vi "Visualize_R&V_Refactored.vi"() -> ()   [LabVIEW 2016]
uses:
  <vilib>/Utility/miscctls.llb/LVPointDoubleTypeDef.ctl
  subVI/DataVIS_StateWire.ctl
panel:
  in  "Decimate Controls 2":T1={"X Low"=-0.1, "X High"=0.1, "X Step"=4e-05, "Voffset -2T"=0.0} {"X Step" format="%#_6p"; "X High" format="%#_6p"; "X Low" format="%#_6p"}
  in  "Decimate Controls":T1={"X Low"=-0.1, "X High"=0.1, "X Step"=4e-05, "Voffset -2T"=0.0} {"X Step" format="%#_6p"; "X High" format="%#_6p"; "X Low" format="%#_6p"}
  in  "Voffset - 2T":dbl format="%#_13g"
  out "Vsd vs Vsg":cluster{dbl[], dbl[]}(graph)
  out "Intensity Graph 12":dbl[][](graph)
  in  "file path (use dialog) 2":path=path "B:/SketchSET/SA03008H.20180718/processed/decimated_21-BG+SG_Sweep+OVERNIGHT"
  out "slowest 2":dbl=4.2894631624221803e-07
  out "Scan names 3":string[](array[string])=["DSA_Vsg1", "B", "B"]
  in  "stop 2":bool
  out "Vfast index":dbl=3.0
  out "Vslow index":i32
  out "side points 4Ttemp 2":i32=8
  out "side points 2Ttemp 2":i32=12
  in  "side points 4T 3":i32=8
  in  "side points 2T 3":i32=12
  in  "Fit Points 3":dbl=10.0
  in  "T/B     third axis 2":bool
  in  "color scale 2":u32[](array[colorbox])=[16711680, 16772608, 6618880, 3381759, 16860, 10420479]
  in  "Voffset -2T 2":dbl=2e-05 format="%#_6p"
  in  "Voffset-4T 2":dbl=-5e-05 format="%#_4p"
  in  "Filter retrieved data?":bool=TRUE
  in  "Field/Temperature 2":i32(slide) min=0 max=36 step=1
  in  "Generate (T) or Visualize (F)":bool
  in  "Tab Control":T2(tab)=enum."3D"
  out "Comments":string="      #Vslow/#Vfast/# of IV curves/BT offset/#discarded IV curves/Manual offset:\n /101/41/1/0/0/0    \n#of fields: 1    \nField period 1 \nDecimate point 10.000000 \nScan names \nDSA_Vsg1\nB\nB \n IGOR\nX// Date: 7/19/2018 7:21 AM\nX// SA03008H\nX// \nX// Source 2 Drain 28 (lockin 1 and 7)\nX// Slow sweeping BG -5 to 5 inc. 0.1V \nX// Fast sweep SG -1 to 1 inc. 0.05V\n\nX// DSA_Vsg1=1.000000\n\nX// \nX// B= 0.000000\n\n\n\n\n\n\n\n\n\n\n\n\n\n\n\n\n\n\n\n\n\n\n\n\n\n\n\n\n\n\n\n\n\n\n\n\n\n\n\n\nX \nX Display/R 'time.SA03008H.20180718.004140'\nX AppendToGraph 'temp.SA03008H.20180718.004140'\nX AppendToGraph 'B.SA03008H.20180718.004140'\nX AppendToGraph 'Vsource.SA03008H.20180718.004140'\nX AppendToGraph 'Lockin0.SA03008H.20180718.004140'\nX AppendToGraph 'Lockin1.SA03008H.20180718.004140'\nX AppendToGraph 'Lockin2.SA03008H.20180718.004140'\nX AppendToGraph 'Lockin3.SA03008H.20180718.004140'\nX AppendToGraph 'Lockin4.SA03008H.20180718.004140'\nX AppendToGraph 'Lockin5.SA03008H.20180718.004140'\nX AppendToGraph 'B_rate.SA03008H.20180718.004140'\nX AppendToGraph 'DC0.SA03008H.20180718.004140'\nX AppendToGraph 'DC1.SA03008H.20180718.004140'\nX AppendToGraph 'DC2.SA03008H.20180718.004140'\nX AppendToGraph 'DC3.SA03008H.20180718.004140'\nX AppendToGraph 'DC4.SA03008H.20180718.004140'\nX AppendToGraph 'DC5.SA03008H.20180718.004140'\nX AppendToGraph 'DC6.SA03008H.20180718.004140'\nX AppendToGraph 'DC7.SA03008H.20180718.004140'\nX Label bottom \"x label\"\nX Label left \"y label\"\nX ModifyGraph rgb('time.SA03008H.20180718.004140')=(65280,0,0)\nX ModifyGraph rgb('temp.SA03008H.20180718.004140')=(65280,18432,0)\nX ModifyGraph rgb('B.SA03008H.20180718.004140')=(65280,36864,0)\nX ModifyGraph rgb('Vsource.SA03008H.20180718.004140')=(65280,55296,0)\nX ModifyGraph rgb('Lockin0.SA03008H.20180718.004140')=(57344,65280,0)\nX ModifyGraph rgb('Lockin1.SA03008H.20180718.004140')=(37376,65280,0)\nX ModifyGraph rgb('Lockin2.SA03008H.20180718.004140')=(18944,65280,0)\nX ModifyGraph rgb('Lockin3.SA03008H.20180718.004140')=(512,65280,0)\nX ModifyGraph rgb('Lockin4.SA03008H.20180718.004140')=(0,65280,17920)\nX ModifyGraph rgb('Lockin5.SA03008H.20180718.004140')=(0,65280,36352)\nX ModifyGraph rgb('B_rate.SA03008H.20180718.004140')=(0,65280,54784)\nX ModifyGraph rgb('DC0.SA03008H.20180718.004140')=(0,57856,65280)\nX ModifyGraph rgb('DC1.SA03008H.20180718.004140')=(0,39424,65280)\nX ModifyGraph rgb('DC2.SA03008H.20180718.004140')=(0,20992,65280)\nX ModifyGraph rgb('DC3.SA03008H.20180718.004140')=(0,2560,65280)\nX ModifyGraph rgb('DC4.SA03008H.20180718.004140')=(17408,0,65280)\nX ModifyGraph rgb('DC5.SA03008H.20180718.004140')=(35840,0,65280)\nX ModifyGraph rgb('DC6.SA03008H.20180718.004140')=(54272,0,65280)\nX ModifyGraph rgb('DC7.SA03008H.20180718.004140')=(65280,0,58368)\nX Legend/C/N=text0/J \"\\\\s('time.SA03008H.20180718.004140') time\\r\\\\s('temp.SA03008H.20180718.004140') temp\\r\\\\s('B.SA03008H.20180718.004140') B\\r\\\\s('Vsource.SA03008H.20180718.004140') Vsource\\r\\\\s('Lockin0.SA03008H.20180718.004140') Lockin0\\r\\\\s('Lockin1.SA03008H.20180718.004140') Lockin1\\r\\\\s('Lockin2.SA03008H.20180718.004140') Lockin2\\r\\\\s('Lockin3.SA03008H.20180718.004140') Lockin3\\r\\\\s('Lockin4.SA03008H.20180718.004140') Lockin4\\r\\\\s('Lockin5.SA03008H.20180718.004140') Lockin5\\r\\\\s('B_rate.SA03008H.20180718.004140') B_rate\\r\\\\s('DC0.SA03008H.20180718.004140') DC0\\r\\\\s('DC1.SA03008H.20180718.004140') DC1\\r\\\\s('DC2.SA03008H.20180718.004140') DC2\\r\\\\s('DC3.SA03008H.20180718.004140') DC3\\r\\\\s('DC4.SA03008H.20180718.004140') DC4\\r\\\\s('DC5.SA03008H.20180718.004140') DC5\\r\\\\s('DC6.SA03008H.20180718.004140') DC6\\r\\\\s('DC7.SA03008H.20180718.004140') DC7\"\nX ModifyGraph mirror(bottom)=1\nX ModifyGraph width=216\nX ModifyGraph height={Aspect,0.6}\nX ModifyGraph Log(bottom)=0\nX ModifyGraph Log(left)=0\nX \n"
  in  "Additional comments":string
  in  "Field Period":i32=1
  in  "# of fields/Temperatures":i32=1
  in  "File or Folder Path":path=path "B:/SketchSET/SA03008H.20180718/21-BG+SG_Sweep+OVERNIGHT"
  in  "Processed data folder":path=path "B:/SketchSET/SA03008H.20180718/processed"
  in  "IV file name":string="decimated_21-BG+SG_Sweep+OVERNIGHT"
  in  "IV setup":T3={"# of Vslow"=101, "# Vfast"=41, "#IV Curves at each gate"=1, "B/T offset"=0, "Discard first # curves"=0, "Manual offset"=0}
  in  "Scan names 2":string[](array[string])=["DSA_Vsg1", "B", "B"]
  in  "Portion of data":cluster{dbl, dbl}(slide)={1.0, 0.0} scale=0.0..1.0
  in  "Decimate point":dbl=10.0 format="%#_1f"
  in  "Extract parameters from comments?":bool=TRUE
  in  "index 2":T4={"A"=3, "B"=5, "C"=3, "D"=5, "E"=3, "N1"=2, "N2"=2, "N3"=3, "N4"=4, "A 1"=3, "A 2"=3, "C 1"=3, "C 2"=3, "E 2"=4}
  out "dV/dI 2T":cluster{dbl[], dbl[]}[](graph)
  out "dV/dI vs I":cluster{dbl[], dbl[]}[](graph)
  out "IV 2T":cluster{dbl[], dbl[]}[](graph)
  out "dI/dV 2T":cluster{dbl[], dbl[]}[](graph)
  out "dI/dV vs V":cluster{dbl[], dbl[]}[](graph)
  out "IV":cluster{dbl[], dbl[]}[](graph)
  out "IV slow 2T":cluster{dbl[], dbl[]}[](graph)
  out "dI/dV slow 2T":cluster{dbl[], dbl[]}[](graph)
  out "IV slow 4T":cluster{dbl[], dbl[]}[](graph)
  out "dI/dV slow 4T":cluster{dbl[], dbl[]}[](graph)
  out "IV vary 3rd 2T":cluster{dbl[], dbl[]}[](graph)
  out "dI/dV vary 3rd 2T":cluster{dbl[], dbl[]}[](graph)
  out "IV vary 3rd 4T":cluster{dbl[], dbl[]}[](graph)
  out "dI/dV vary 3rd 4T":cluster{dbl[], dbl[]}[](graph)
  out "X line cut 2":cluster{dbl[], dbl[]}(graph)
  out "Y line cut 2":cluster{dbl[], dbl[]}(graph)={[-1.0, -0.95, -0.9, -0.85, -0.8, -0.75, -0.7, -0.65, -0.6, -0.55, -0.5, -0.45, -0.4, -0.35, -0.3, -0.25, -0.2, -0.15, -0.1, -0.05, 0.0, 0.05, 0.1, 0.15, 0.2, 0.25, 0.3, 0.35, 0.4, 0.45, 0.5, 0.55, 0.6, 0.65, 0.7, 0.75, 0.8, 0.85, 0.9, 0.95, 1.0], [0.0, 0.0, 0.0, 0.0, 0.0, 0.0, 0.0, 0.0, 0.0, 0.0, 0.0, 0.0, 0.0, 0.0, 0.0, 0.0, 0.0, 0.0, 0.0, 0.0, 0.0, 0.0, 0.0, 0.0, 0.0, 0.0, 0.0, 0.0, 0.0, 0.0, 0.0, 0.0, 0.0, 0.0, 0.0, 0.0, 0.0, 0.0, 0.0, 0.0, 0.0]}
  out "Intensity Graph":dbl[][](graph)
  out "Intensity Graph 2":dbl[][](graph)
  in  "X Low":dbl=-0.1 format="%#_6p"
  in  "X High":dbl=0.1 format="%#_6p"
  in  "X Step":dbl=5e-05 format="%#_6p"
  in  "Log scale? 2":bool
  in  "Log scale?":bool
  in  "No scale?":bool
  in  "Breakdown Low":dbl=-0.1 format="%#_6p"
  in  "Breakdown High":dbl=0.2 format="%#_6p"
  out "X scale":cluster{dbl, "X Step":dbl}={-0.09995000000000001, "X Step"=5e-05}
  out "Y scale":cluster{"Real Voltage":dbl, dbl}={"Real Voltage"=-1.0, 0.050000000000000044}
  in  "fake point value":dbl format="%#_6p"
  out "Transconductance":dbl[][](graph)
  in  "derivative bin size (also for 2T)":dbl=15.0
  out "Field 2":dbl=-3.687258687258687
  out "X line cut 3":cluster{dbl[], dbl[]}(graph)
  out "X line cut 7":cluster{dbl[], dbl[]}(graph)={array[399 elements], [-0.0, -0.0, -0.0, -0.0, -0.0, -0.0, -0.0, -0.0, -0.0, -0.0, -0.0, -0.0, -0.0, -0.0, -0.0, -0.0, -0.0, -0.0, -0.0, -0.0, -0.0, -0.0, -0.0, -0.0, -0.0, -0.0, -0.0, -0.0, -0.0, -0.0, -0.0, -0.0, -0.0, -0.0, -0.0, -0.0, -0.0, -0.0, -0.0, -0.0, -0.0, -0.0, -0.0, -0.0, -0.0, -0.0, -0.0, -0.0, -0.0, -0.0, -0.0, -0.0, -0.0, -0.0, -0.0, -0.0, -0.0, -0.0, -0.0, -0.0, -0.0, -0.0, -0.0, -0.0, -0.0, -0.0, -0.0, -0.0, -0.0, -0.0, -0.0, -0.0, -0.0, -0.0, -0.0, -0.0, -0.0, -0.0, -0.0, -0.0, -0.0, -0.0, -0.0, -0.0, -0.0, -0.0, -0.0, -0.0, -0.0, -0.0, -0.0, -0.0, -0.0, -0.0, -0.0, -0.0, -0.0, -0.0, -0.0, -0.0, -0.0, -0.0, -0.0, -0.0, -0.0, -0.0, -0.0, -0.0, -0.0, -0.0, -0.0, -0.0, -0.0, -0.0, -0.0, -0.0, -0.0, -0.0, -0.0, -0.0, -0.0, -0.0, -0.0, -0.0, -0.0, -0.0, -0.0, -0.0, -0.0, -0.0, -0.0, -0.0, -0.0, -0.0, -0.0, -0.0, -0.0, -0.0, -0.0, -0.0, -0.0, -0.0, -0.0, -0.0, -0.0, -0.0, -0.0, -0.0, -0.0, -0.0, -0.0, -0.0, -0.0, -0.0, -0.0, -0.0, -0.0, -0.0, -0.0, -0.0, -0.0, -0.0, -0.0, -0.0, -0.0, -0.0, -0.0, -0.0, -0.0, -0.0, -0.0, -0.0, -0.0, -0.0, -0.0, -0.0, -0.0, -0.0, -0.0, -0.0, -0.0, -0.0, -0.0, -0.0, -0.0, -0.0, -0.0, -0.0, -0.0, -0.0, -0.0, -0.0, -0.0, -0.0, -0.0, -0.0, -0.0, -0.0, -0.0, -0.0, -0.0, -0.0, -0.0, -0.0, -0.0, -0.0, -0.0, -0.0, -0.0, -0.0, -0.0, -0.0, -0.0, -0.0, -0.0, -0.0, -0.0, -0.0, -0.0, -0.0, -0.0, -0.0, -0.0, -0.0, -0.0, -0.0, -0.0, -0.0, -0.0, -0.0, -0.0, -0.0, -0.0, -0.0, -0.0, -0.0, -0.0, -0.0, -0.0, -0.0, -0.0, -0.0, -0.0, -0.0, -0.0, -0.0, -0.0, -0.0, -0.0, -0.0, -0.0, -0.0, -0.0, -0.0, -0.0, -0.0, -0.0, -0.0, -0.0, -0.0, -0.0, -0.0, -0.0, -0.0, -0.0, -0.0, -0.0, -0.0, -0.0, -0.0, -0.0, -0.0, -0.0, -0.0, -0.0, -0.0, -0.0, -0.0, -0.0, -0.0, -0.0, -0.0, -0.0, -0.0, -0.0, -0.0, -0.0, -0.0, -0.0, -0.0, -0.0, -0.0, -0.0, -0.0, -0.0, -0.0, -0.0, -0.0, -0.0, -0.0, -0.0, -0.0, -0.0, -0.0, -0.0, -0.0, -0.0, -0.0, -0.0, -0.0, -0.0, -0.0, -0.0, -0.0, -0.0, -0.0, -0.0, -0.0, -0.0, -0.0, -0.0, -0.0, -0.0, -0.0, -0.0, -0.0, -0.0, -0.0, -0.0, -0.0, -0.0, -0.0, -0.0, -0.0, -0.0, -0.0, -0.0, -0.0, -0.0, -0.0, -0.0, -0.0, -0.0, -0.0, -0.0, -0.0, -0.0, -0.0, -0.0, -0.0, -0.0, -0.0, -0.0, -0.0, -0.0, -0.0, -0.0, -0.0, -0.0, -0.0, -0.0, -0.0, -0.0, -0.0, -0.0, -0.0, -0.0, -0.0, -0.0, -0.0, -0.0, -0.0, -0.0, -0.0, -0.0, -0.0, -0.0, -0.0, -0.0, -0.0, -0.0, -0.0, -0.0, -0.0, -0.0, -0.0, -0.0, -0.0, -0.0, -0.0, -0.0, -0.0, -0.0, -0.0, -0.0, -0.0, -0.0, -0.0, -0.0]}
  out "Y line cut 8":cluster{dbl[], dbl[]}(graph)={[-1.0, -0.95, -0.9, -0.85, -0.8, -0.75, -0.7, -0.65, -0.6, -0.55, -0.5, -0.45, -0.4, -0.35, -0.3, -0.25, -0.2, -0.15, -0.1, -0.05, 0.0, 0.05, 0.1, 0.15, 0.2, 0.25, 0.3, 0.35, 0.4, 0.45, 0.5, 0.55, 0.6, 0.65, 0.7, 0.75, 0.8, 0.85, 0.9, 0.95, 1.0], [-0.0, -0.0, -0.0, -0.0, -0.0, -0.0, -0.0, -0.0, -0.0, -0.0, -0.0, -0.0, -0.0, -0.0, -0.0, -0.0, -0.0, -0.0, -0.0, -0.0, -0.0, -0.0, -0.0, -0.0, -0.0, -0.0, -0.0]}
  out "Y line cut":cluster{"Vfast":dbl[], dbl[]}(graph)
  out "X line cut":cluster{dbl[], dbl[]}(graph)
  out "2 term trans":dbl[][](graph)
  in  "X Step 2T":dbl=4e-05 format="%#_6p"
  in  "X High 2T":dbl=0.1 format="%#_6p"
  in  "X Low 2T":dbl=-0.1 format="%#_6p"
  in  "Log scale? 4":bool
  in  "Log scale? 3":bool
  out "2term Intensity 2":dbl[][](graph)
  in  "fake point value 2":dbl format="%#_6p"
  out "2term trans X line cut":cluster{dbl[], dbl[]}(graph)
  out "2term trans Y line cut":cluster{"Vfast":dbl[], dbl[]}(graph)
  in  "e^2/h?":bool
  out "2term Intensity Current vs. Voltage":dbl[][](graph)
  in  "width X 6":dbl=1e-09 min=1.0 format="%#_6p"
  in  "width Y 6":dbl=1e-09 min=1.0 format="%#_6p"
  out "Y line cut 6":cluster{"Vfast":dbl[], dbl[]}(graph)={"Vfast"=[-5.0, -4.9, -4.8, -4.7, -4.6, -4.5, -4.4, -4.3, -4.2, -4.1, -4.0, -3.9, -3.8, -3.7, -3.5999999999999996, -3.5, -3.4, -3.3, -3.2, -3.0999999999999996, -3.0, -2.9, -2.8, -2.6999999999999997, -2.5999999999999996, -2.5, -2.4, -2.3, -2.1999999999999997, -2.0999999999999996, -2.0, -1.9, -1.7999999999999998, -1.6999999999999997, -1.5999999999999996, -1.5, -1.4, -1.2999999999999998, -1.1999999999999997, -1.0999999999999996, -1.0, -0.8999999999999995, -0.7999999999999998, -0.7000000000000002, -0.5999999999999996, -0.5, -0.39999999999999947, -0.2999999999999998, -0.1999999999999993, -0.09999999999999964, 0.0, 0.10000000000000053, 0.20000000000000018, 0.3000000000000007, 0.40000000000000036, 0.5, 0.6000000000000005, 0.7000000000000002, 0.8000000000000007, 0.9000000000000004, 1.0, 1.1000000000000005, 1.2000000000000002, 1.3000000000000007, 1.4000000000000004, 1.5, 1.6000000000000005, 1.7000000000000002, 1.8000000000000007, 1.9000000000000004, 2.0, 2.1000000000000005, 2.2, 2.3000000000000007, 2.4000000000000004, 2.5, 2.6000000000000005, 2.7, 2.8000000000000007, 2.9000000000000004, 3.0, 3.0999999999999996, 3.200000000000001, 3.3000000000000007, 3.4000000000000004, 3.5, 3.5999999999999996, 3.700000000000001, 3.8000000000000007, 3.9000000000000004, 4.0, 4.1, 4.200000000000001, 4.300000000000001, 4.4, 4.5, 4.600000000000001, 4.700000000000001, 4.800000000000001, 4.9, 5.0], [0.02727272727272727, 0.02727272727272727, 0.02727272727272727, 0.02727272727272727, 0.02727272727272727, 0.02727272727272727, 0.02727272727272727, 0.02727272727272727, 0.02727272727272727, 0.02727272727272727, 0.02727272727272727, 0.02727272727272727, 0.02727272727272727, 0.02727272727272727, 0.02727272727272727, 0.02727272727272727, 0.02727272727272727, 0.02727272727272727, 0.02727272727272727, 0.02727272727272727, 0.02727272727272727, 0.02727272727272727, 0.02727272727272727, 0.02727272727272727, 0.02727272727272727, 0.02727272727272727, 0.02727272727272727, 0.02727272727272727, 0.02727272727272727, 0.02727272727272727, 0.02727272727272727, 0.02727272727272727, 0.02727272727272727, 0.02727272727272727, 0.02727272727272727, 0.02727272727272727, 0.02727272727272727, 0.02727272727272727, 0.02727272727272727, 0.02727272727272727, 0.02727272727272727, 0.02727272727272727, 0.02727272727272727, 0.02727272727272727, 0.02727272727272727, 0.02727272727272727, 0.02727272727272727, 0.02727272727272727, 0.02727272727272727, 0.02727272727272727, 0.02727272727272727, 0.02727272727272727, 0.02727272727272727, 0.02727272727272727, 0.02727272727272727, 0.02727272727272727, 0.02727272727272727, 0.02727272727272727, 0.02727272727272727, 0.02727272727272727, 0.02727272727272727, 0.02727272727272727, 0.02727272727272727, 0.02727272727272727, 0.02727272727272727, 0.02727272727272727, 0.02727272727272727, 0.02727272727272727, 0.02727272727272727, 0.02727272727272727, 0.02727272727272727, 0.02727272727272727, 0.02727272727272727, 0.02727272727272727, 0.02727272727272727, 0.02727272727272727, 0.02727272727272727, 0.02727272727272727, 0.02727272727272727, 0.02727272727272727, 0.02727272727272727, 0.02727272727272727, 0.02727272727272727, 0.02727272727272727, 0.02727272727272727, 0.02727272727272727, 0.02727272727272727, 0.02727272727272727, 0.02727272727272727, 0.02727272727272727, 0.02727272727272727, 0.02727272727272727, 0.02727272727272727, 0.02727272727272727, 0.02727272727272727, 0.02727272727272727, 0.02727272727272727, 0.02727272727272727, 0.02727272727272727, 0.02727272727272727, 0.02727272727272727]}
  out "X line cut 6":cluster{dbl[], dbl[]}(graph)
  out "Y line cut 5":cluster{"Vfast":dbl[], dbl[]}(graph)={"Vfast"=[-1.0, -0.95, -0.9, -0.85, -0.8, -0.75, -0.7, -0.65, -0.6, -0.55, -0.5, -0.45, -0.4, -0.35, -0.3, -0.25, -0.2, -0.15, -0.1, -0.05, 0.0, 0.05, 0.1, 0.15, 0.2, 0.25, 0.3, 0.35, 0.4, 0.45, 0.5, 0.55, 0.6, 0.65, 0.7, 0.75, 0.8, 0.85, 0.9, 0.95, 1.0], [0.049999999999999996, 0.049999999999999996, 0.049999999999999996, 0.049999999999999996, 0.049999999999999996, 0.049999999999999996, 0.049999999999999996, 0.049999999999999996, 0.049999999999999996, 0.049999999999999996, 0.049999999999999996, 0.049999999999999996, 0.049999999999999996, 0.049999999999999996, 0.049999999999999996, 0.049999999999999996, 0.049999999999999996, 0.049999999999999996, 0.049999999999999996, 0.049999999999999996, 0.049999999999999996, 0.049999999999999996, 0.049999999999999996, 0.049999999999999996, 0.049999999999999996, 0.049999999999999996, 0.049999999999999996, 0.049999999999999996, 0.049999999999999996, 0.049999999999999996, 0.049999999999999996, 0.049999999999999996, 0.049999999999999996, 0.049999999999999996, 0.049999999999999996, 0.049999999999999996, 0.049999999999999996, 0.049999999999999996, 0.049999999999999996, 0.049999999999999996, 0.049999999999999996]}
  out "X line cut 5":cluster{dbl[], dbl[]}(graph)
  out "Intensity Graph 6":dbl[][](graph)
  in  "X Step 4t":dbl=1e-10 format="%#_6p"
  in  "X High 4t":dbl=3e-08 format="%#_6p"
  in  "X Low 4t":dbl=-3e-08 format="%#_6p"
  in  "Log scale? 6":bool
  in  "Log scale? 5":bool
  out "Intensity Graph 5":dbl[][](graph)
  in  "fake point value 3":dbl=0.05 format="%#_6p"
  in  "width X 5":dbl=1e-09 min=1.0 format="%#_6p"
  in  "width Y 5":dbl=1e-09 min=1.0 format="%#_6p"
  out "Y line cut 4":cluster{"Vfast":dbl[], dbl[]}(graph)
  out "X line cut 4":cluster{dbl[], dbl[]}(graph)
  out "Intensity Graph 8":dbl[][](graph)
  in  "X Step 2t":dbl=1e-11 format="%#_6p"
  in  "X High 2t":dbl=1e-09 format="%#_6p"
  in  "X Low 2t":dbl=-2e-09 format="%#_6p"
  in  "Log scale? 8":bool
  in  "Log scale? 7":bool
  out "Intensity Graph 7":dbl[][](graph)
  in  "fake pt value 4":dbl=0.05 format="%#_6p"
  out "Intensity Graph 11":dbl[][](graph)
  out "Intensity Graph 10":dbl[][](graph)
  out "Intensity Graph 9":dbl[][](graph)
  out "Transconductance 2":dbl[][](graph)
  in  "derivative bin size 2":dbl=10.0
  in  "width":i32=3 min=3
  in  "threshold":dbl format="%0.2f"
  out "vertical peak diff":dbl[](array[numeric])
  out "Array 2":dbl[](array[numeric])
  out "Y line cut 9":cluster{dbl[], dbl[]}[](graph)
  in  "width 2":i32=3 min=3
  in  "threshold 2":dbl format="%0.2f"
  in  "calc alpha?":bool
  out "XY Graph 2":cluster{dbl[], dbl[]}(graph)
  in  "Fit Points":dbl=10.0
  out "Field":dbl=-3.687258687258687
  out "slowest":dbl=4.2894631624221803e-07
  in  "Filter retrieved data? 2":bool=TRUE
  in  "stop":bool
  in  "side points 4T 2":i32=8
  out "side points 4Ttemp":i32=8
  in  "side points 2T 2":i32=12
  out "side points 2Ttemp":i32=12
  in  "side points 4T":i32=8
  in  "side points 2T":i32=12
  in  "Fit Points 2":dbl=10.0
  in  "T/B     third axis":bool
  in  "color scale":u32[](array[colorbox])=[16711680, 16772608, 6618880, 3381759, 16860, 10420479]
  in  "Voffset-4T":dbl=-5e-05 format="%#_4p"
  in  "Field/Temperature":i32(slide) min=0 max=36 step=1
  out "Scan names":string[](array[string])=["DSA_Vsg1", "B", "B"]
  in  "file path (use dialog)":path=path "B:/SketchSET/SA03008H.20180718/processed/decimated_21-BG+SG_Sweep+OVERNIGHT"
  in  "OK":bool
  # "VS"
  # "I+"
  # "V+"
  # "Vsg1"
  # "Vsgw"
  # "Vsg2"
  # "V-"
  # "I-"
  # "Output"
  # "Vfast"
  # "Vslow"
  # "Vslowest"
  # "Vfast"
  # "Vslow"
  # "Vslowest"
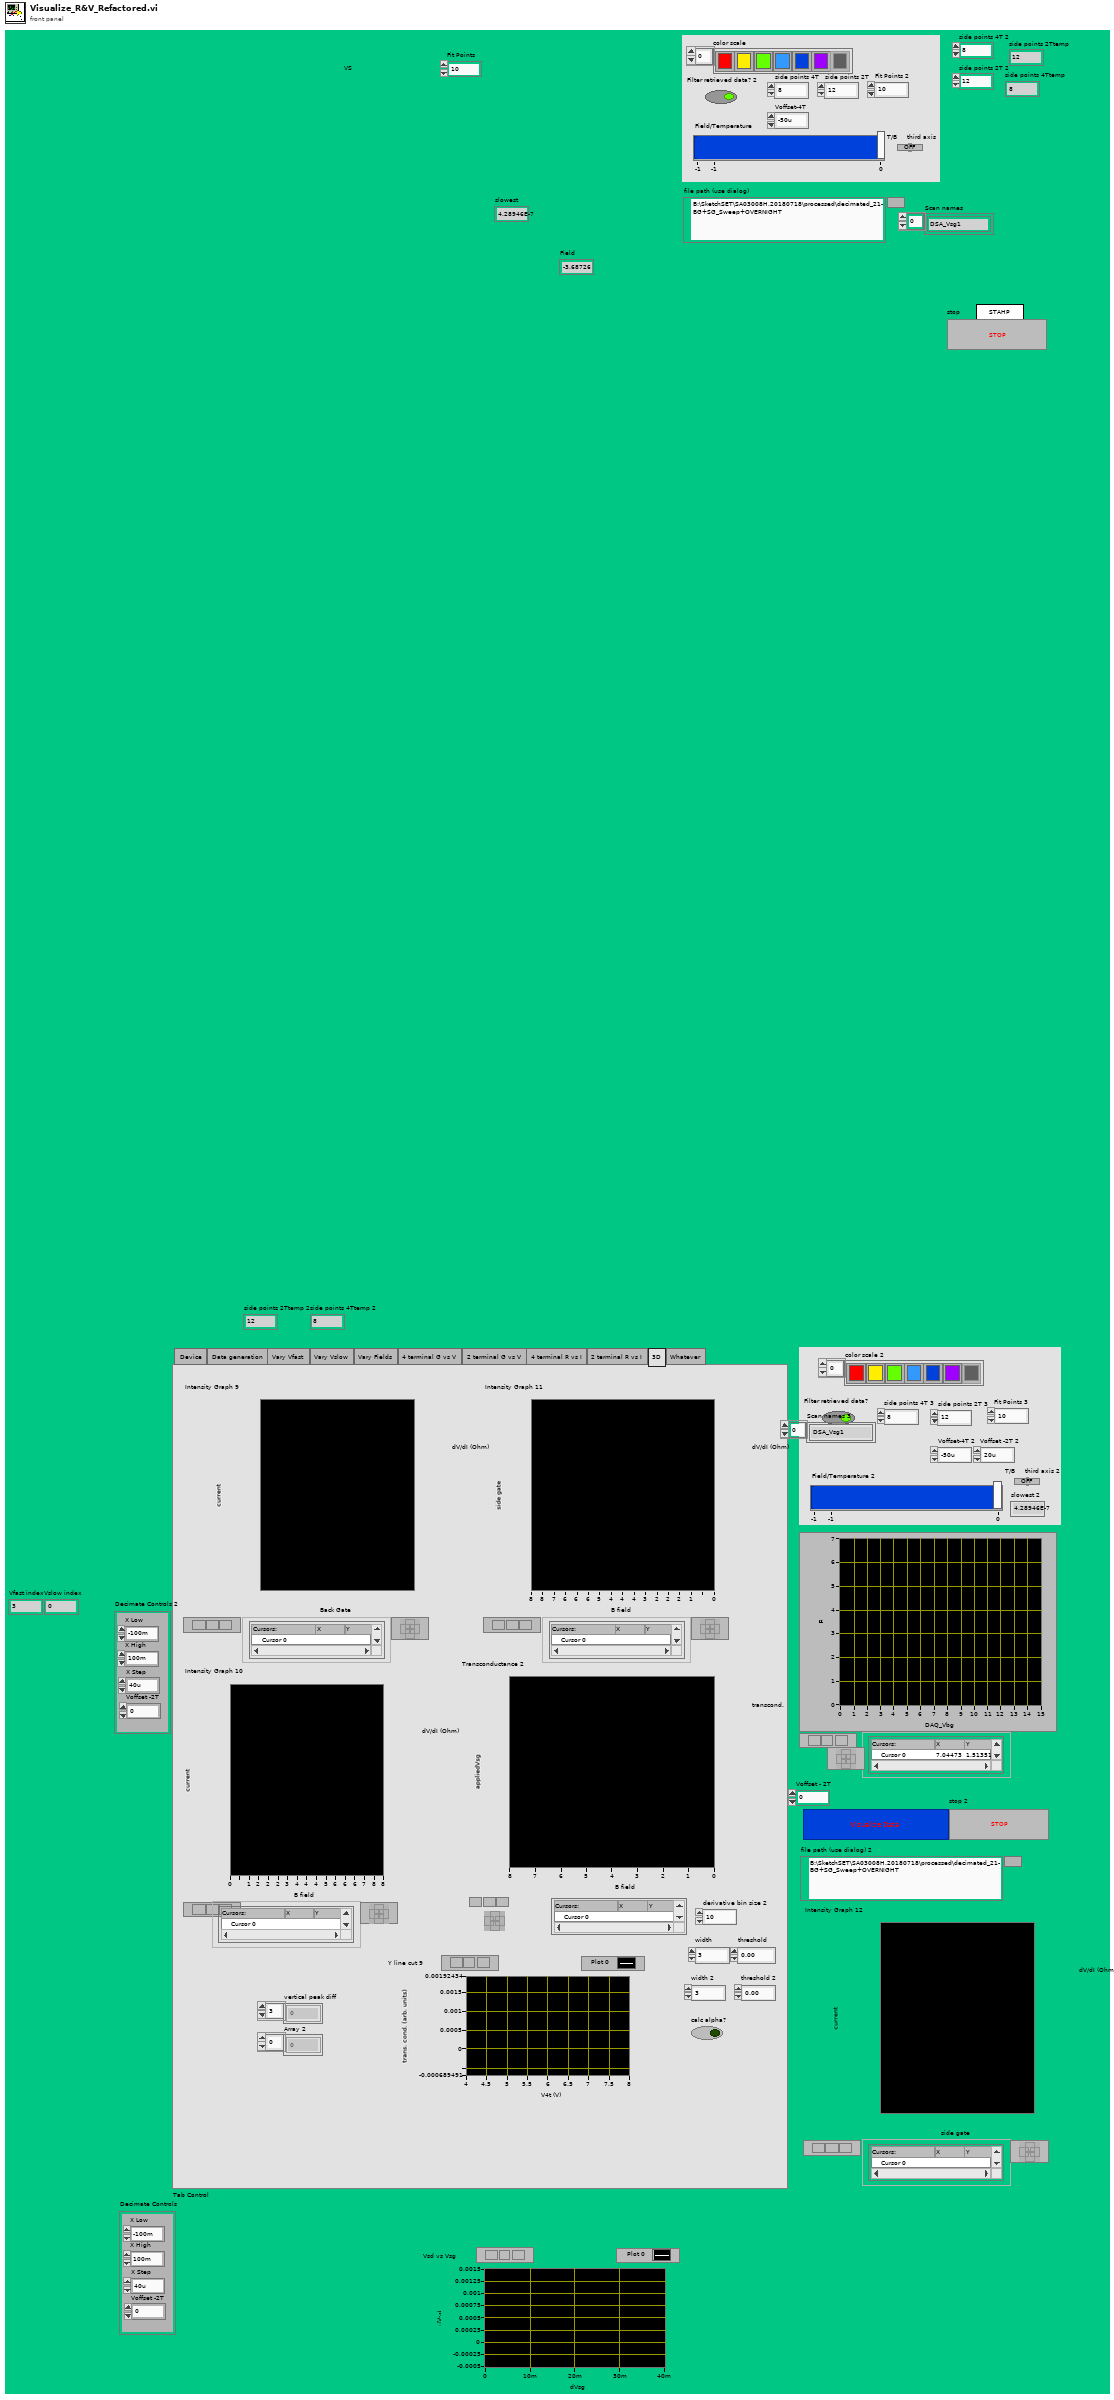
[diagram p1: front panel]
types:
  T1 = cluster{"X Low":dbl, "X High":dbl, "X Step":dbl, "Voffset -2T":dbl}
  T2 = enum32{"Device ", "Data generation", "Vary Vfast", "Vary Vslow", "Vary Fields", "4 terminal G vs V", "2 terminal G vs V", "4 terminal R vs I", "2 terminal R vs I", "3D", "Whatever"}
  T3 = cluster{"# of Vslow":i32, "# Vfast":i32, "#IV Curves at each gate":i32, "B/T offset":i32, "Discard first # curves":i32, "Manual offset":i32}
  T4 = cluster{"A":i32, "B":i32, "C":i32, "D":i32, "E":i32, "N1":i32, "N2":i32, "N3":i32, "N4":i32, "A 1":i32, "A 2":i32, "C 1":i32, "C 2":i32, "E 2":i32}
  T5 = enum32{"invalid app kind", "Development System", "Run Time System", "Student Edition", "Embedded LabVIEW", "Evaluation", "Custom"}
  T6 = enum32{"Invalid", "Standard", "Closed", "Hidden", "Minimized", "Maximized"}
  T7 = typedef "DataVIS_StateWire.ctl" = cluster{"Core":cluster{"Current VI Reference":refnum<vi>, "Close Panel on Exit?":bool}, "data value reference":refnum<data-value>, "Sweep Data Cluster":cluster{"Vfast":dbl[][], "Vslow":dbl[], "Vslowest":dbl[], "Comments":string, "Scan names":string[]}, "Cursor Info":cluster{"Fast Index (Cursor X)":dbl[], "Slow Index (Cursor Y)":dbl, "Slow Indices":dbl[], "Raw Cursor Position":T8, "Field / temp":i32}, "Scan names":string[]}
  T8 = typedef "LVPointDoubleTypeDef.ctl" = cluster{"X":dbl, "Y":dbl}
  T9 = cluster{"Current VI Reference":refnum<vi>, "Close Panel on Exit?":bool}
  T10 = cluster{"Vfast":dbl[][], "Vslow":dbl[], "Vslowest":dbl[], "Comments":string, "Scan names":string[]}
  T11 = cluster{"IV":cluster{dbl[], dbl[]}[][][], "IV-2T":cluster{dbl[], dbl[]}[][][], "Vfast":dbl[][], "Vslow":dbl[], "Vslowest":dbl[], "Comments":string, "Scan names":string[]}[]
  T12 = cluster{"IV":cluster{dbl[], dbl[]}[][][], "IV-2T":cluster{dbl[], dbl[]}[][][], "Vfast":dbl[][], "Vslow":dbl[], "Vslowest":dbl[], "Comments":string, "Scan names":string[]}
  T13 = cluster{"Decimated Array":dbl[], "Decimated Array":dbl[]}
  T14 = cluster{"IV-2T":cluster{dbl[], dbl[]}[][][], "IV":cluster{dbl[], dbl[]}[][][], cluster{"Decimated Array":dbl[], "Decimated Array":dbl[]}[][][], cluster{"Decimated Array":dbl[], "Decimated Array":dbl[]}[][][], cluster{"Decimated Array":dbl[], "Decimated Array":dbl[]}[][][], cluster{"Decimated Array":dbl[], "Decimated Array":dbl[]}[][][]}
  T15 = cluster{"Fast Index (Cursor X)":dbl[], "Slow Index (Cursor Y)":dbl, "Slow Indices":dbl[], "Raw Cursor Position":T8, "Field / temp":i32}
  T16 = cluster{"IV-2T":cluster{dbl[], dbl[]}[][][], "IV":cluster{dbl[], dbl[]}[][][], "dI/dV 2T":cluster{dbl[], dbl[]}[][][], "dV/dI 2T":cluster{dbl[], dbl[]}[][][], "dI/dV vs V":cluster{dbl[], dbl[]}[][][], "dV/dI vs I":cluster{dbl[], dbl[]}[][][]}
  T17 = cluster{"2term Intensity 2":refnum<vi>, "2 term trans":refnum<vi>}
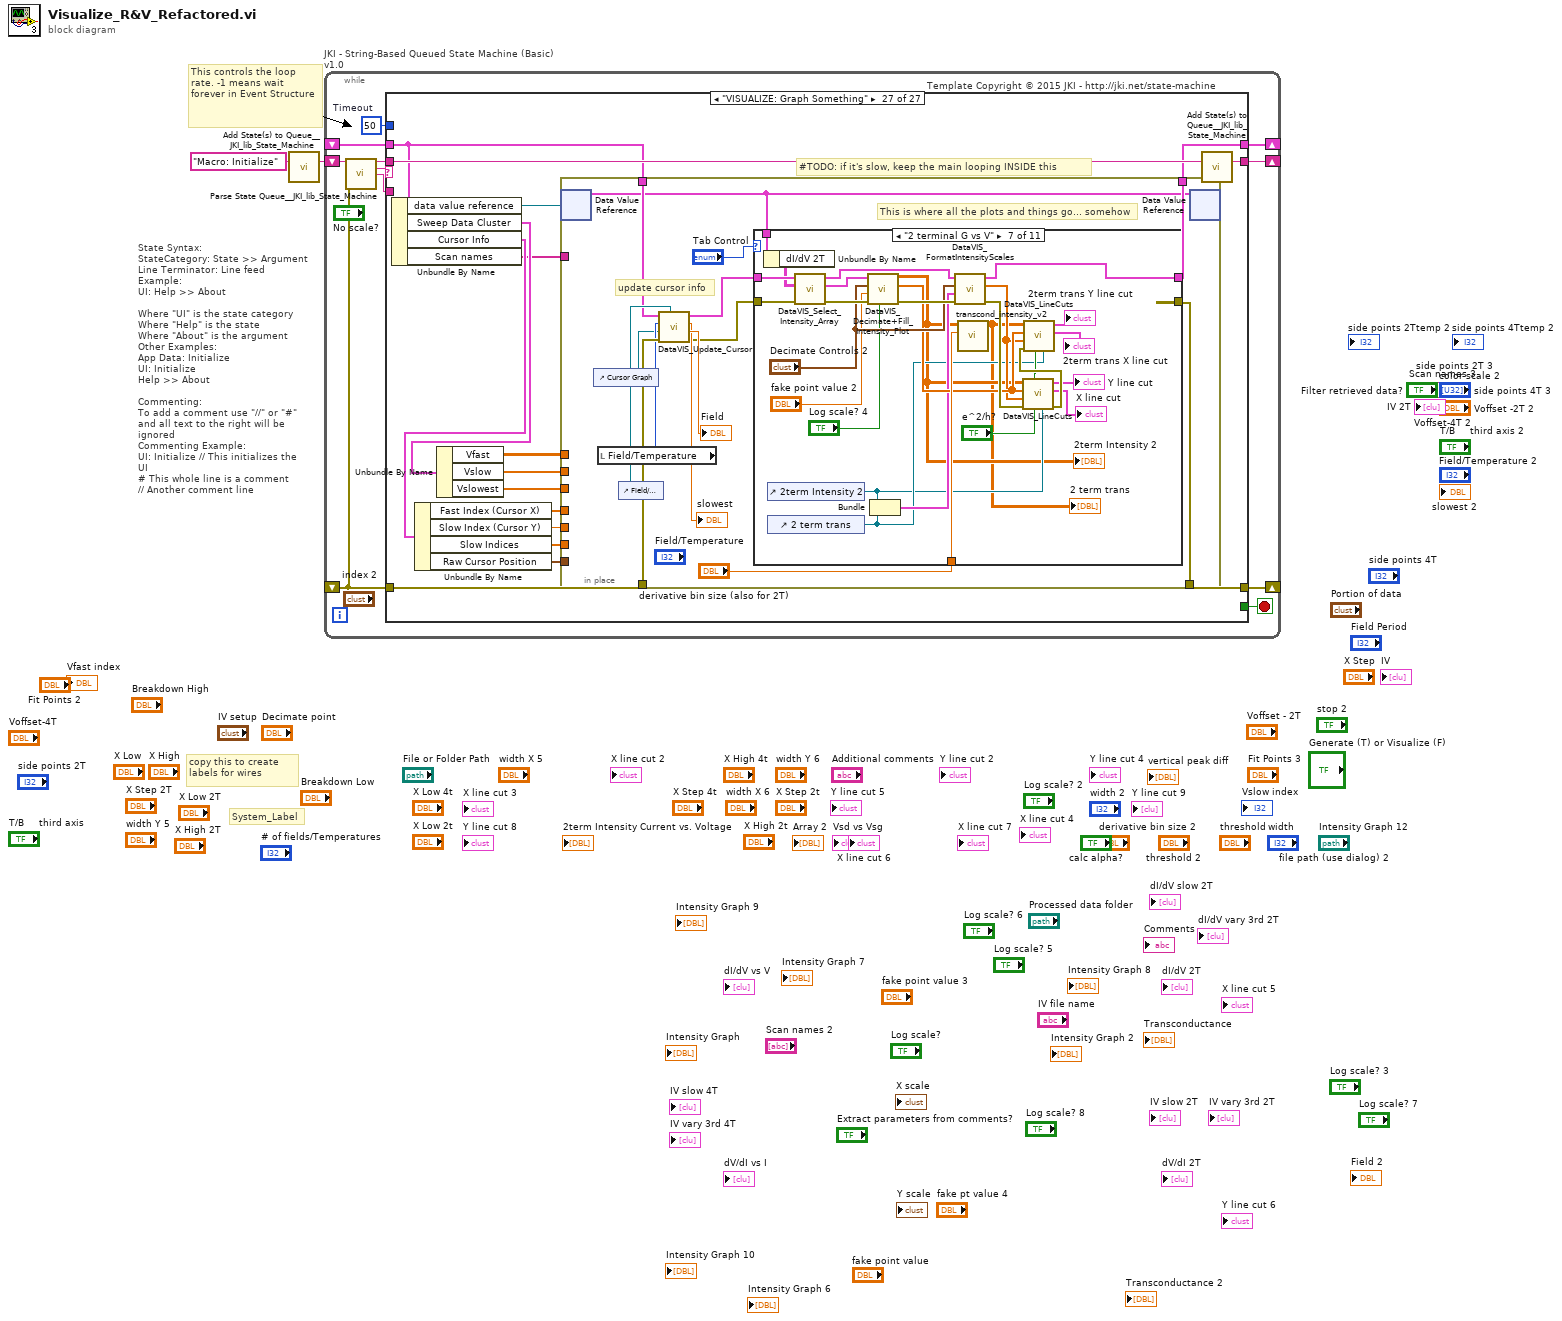
[diagram p0: block diagram]
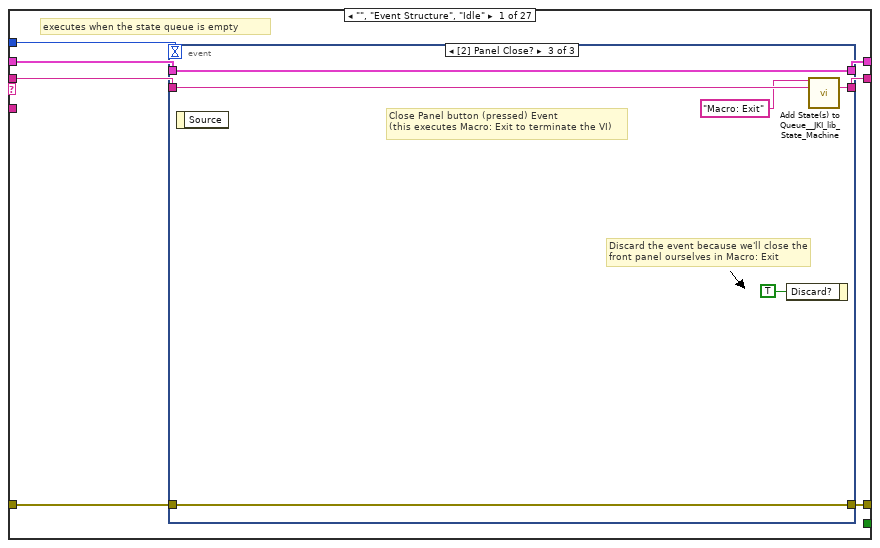
[diagram p2: hidden frame]
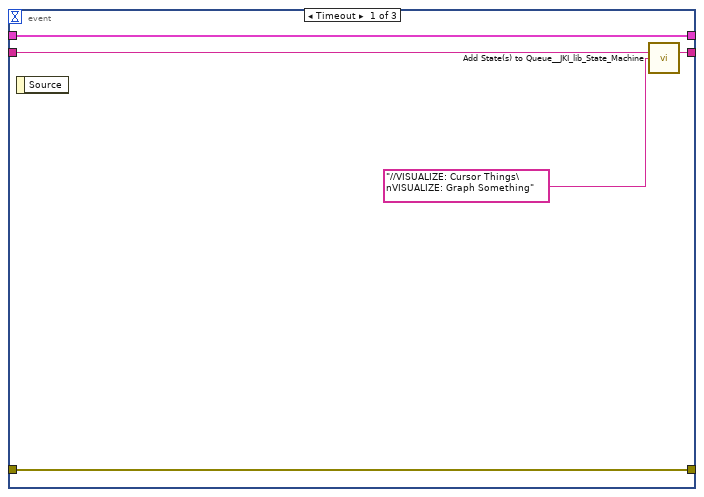
[diagram p3: hidden frame]
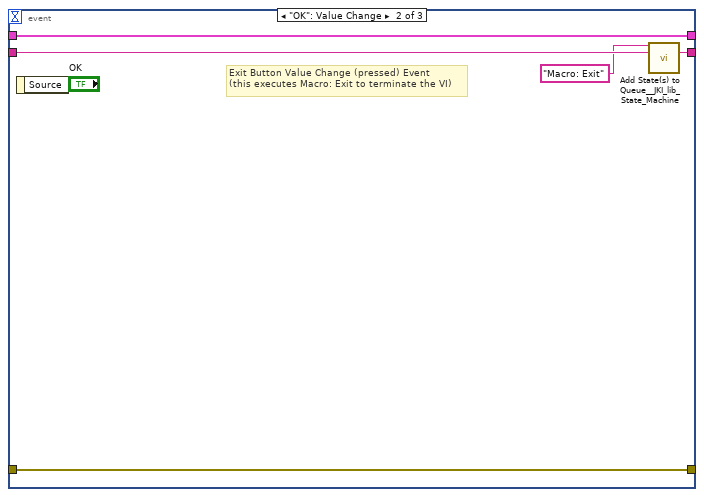
[diagram p4: hidden frame]
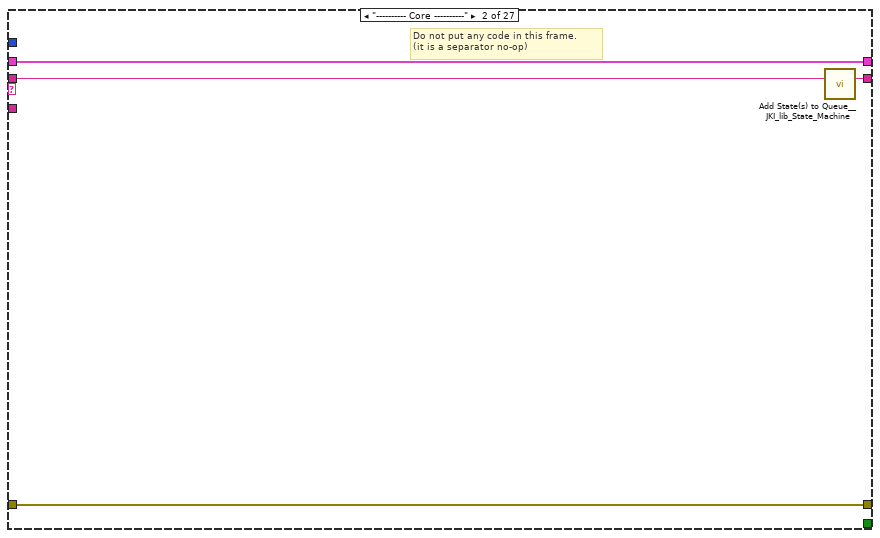
[diagram p5: hidden frame]
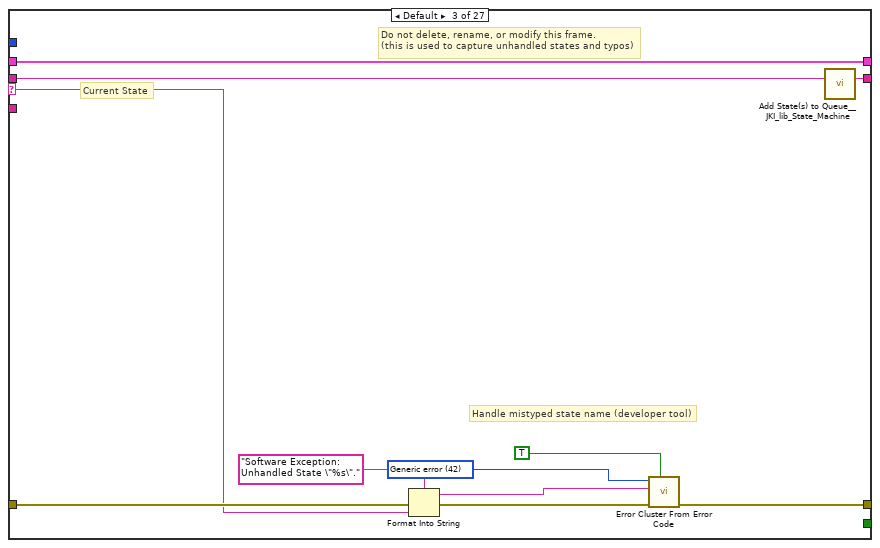
[diagram p6: hidden frame]
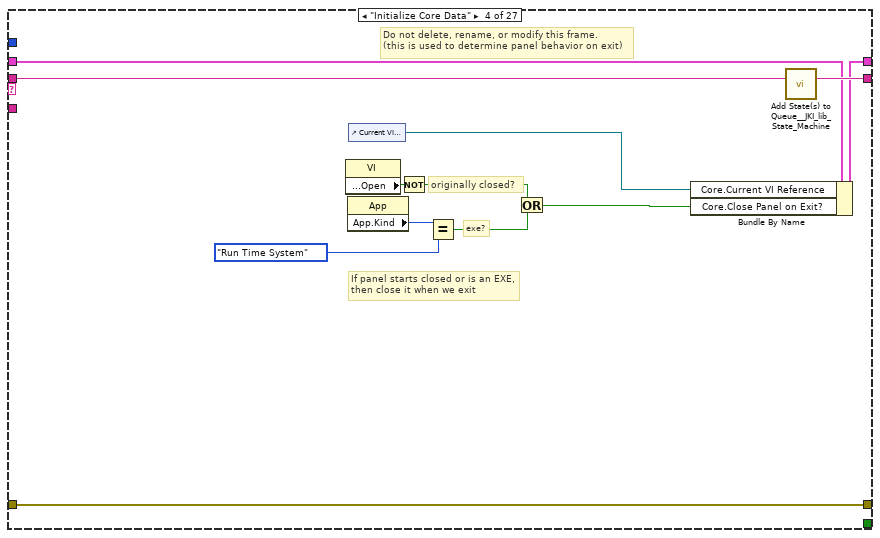
[diagram p7: hidden frame]
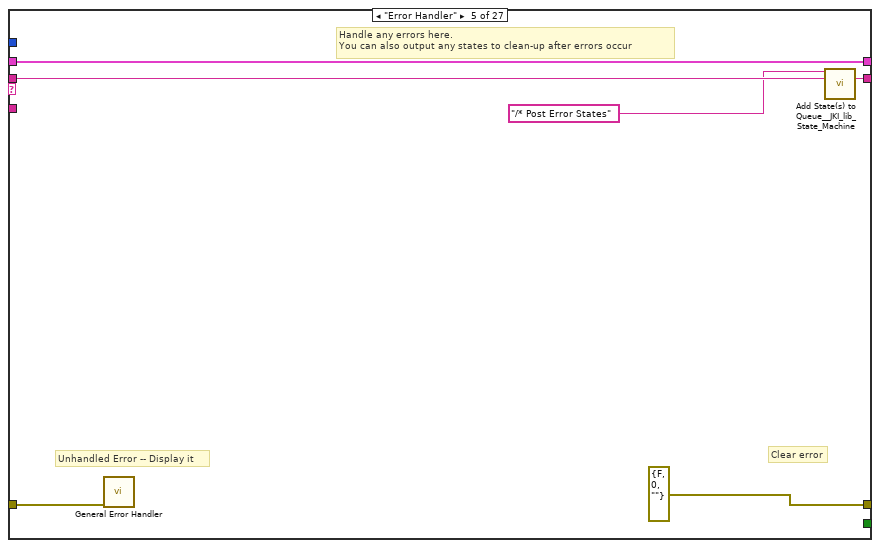
[diagram p8: hidden frame]
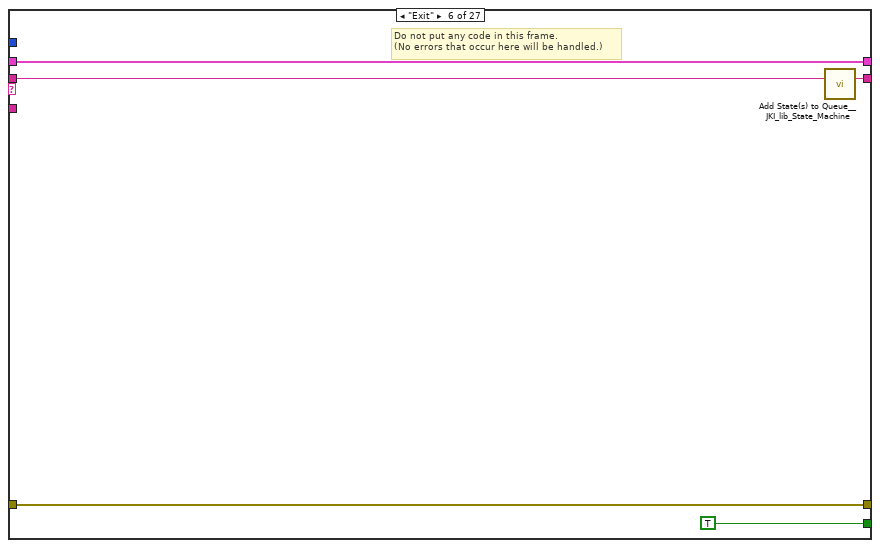
[diagram p9: hidden frame]
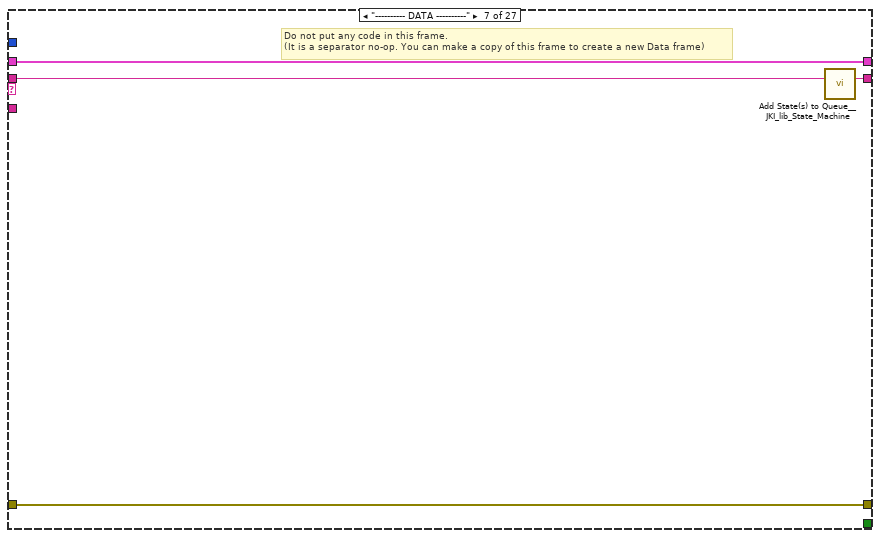
[diagram p10: hidden frame]
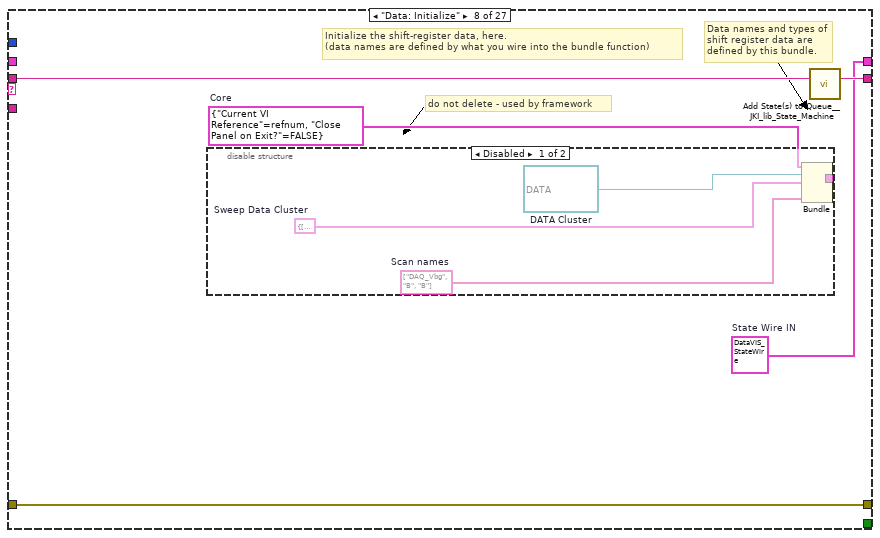
[diagram p11: hidden frame]
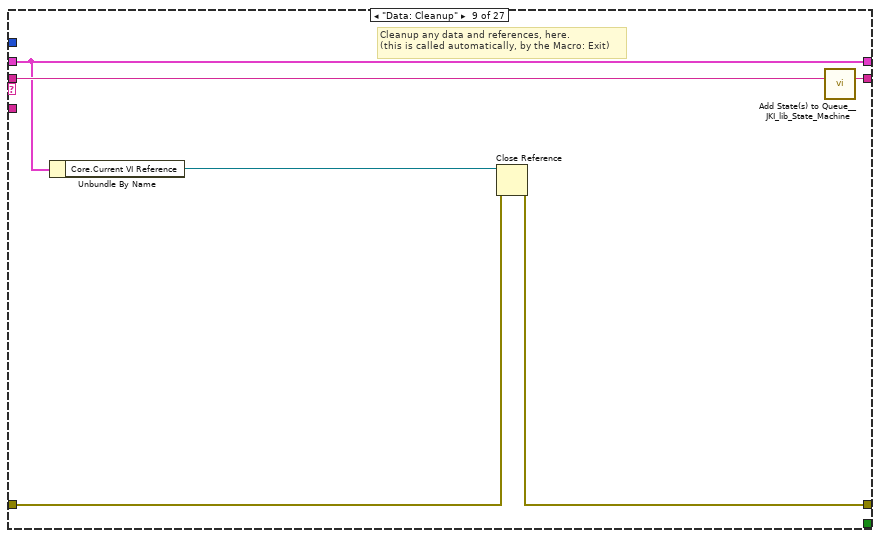
[diagram p13: hidden frame]
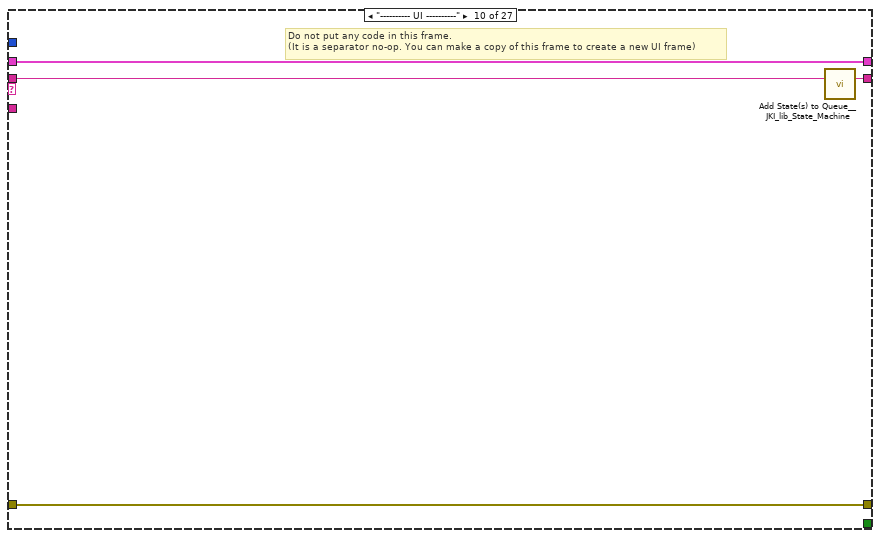
[diagram p14: hidden frame]
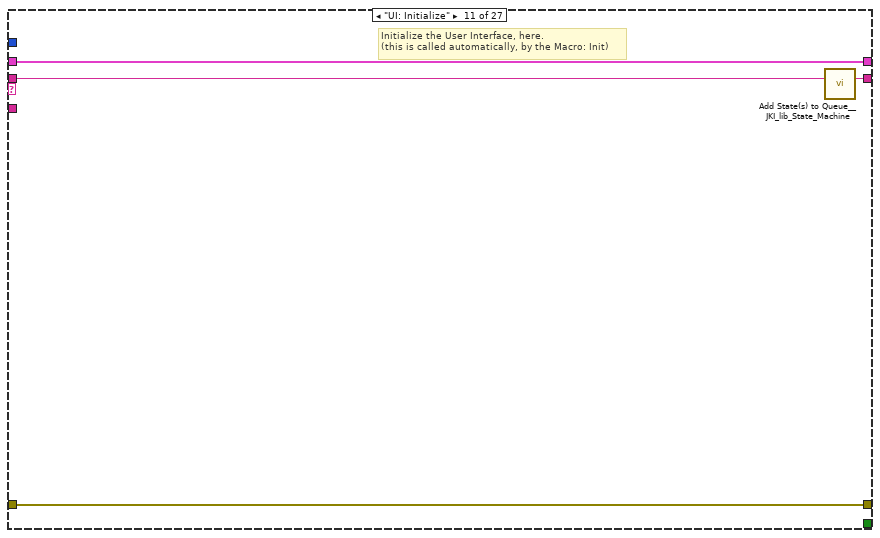
[diagram p15: hidden frame]
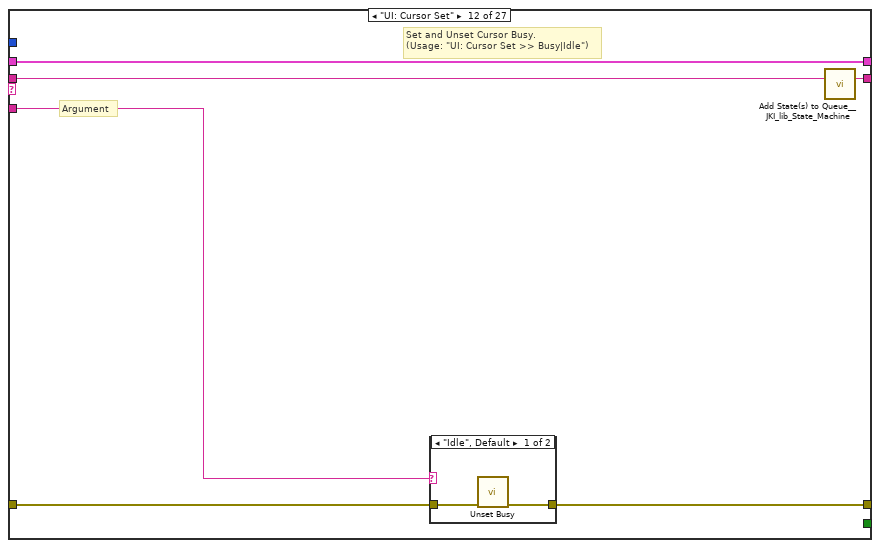
[diagram p16: hidden frame]
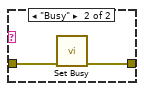
[diagram p17: hidden frame]
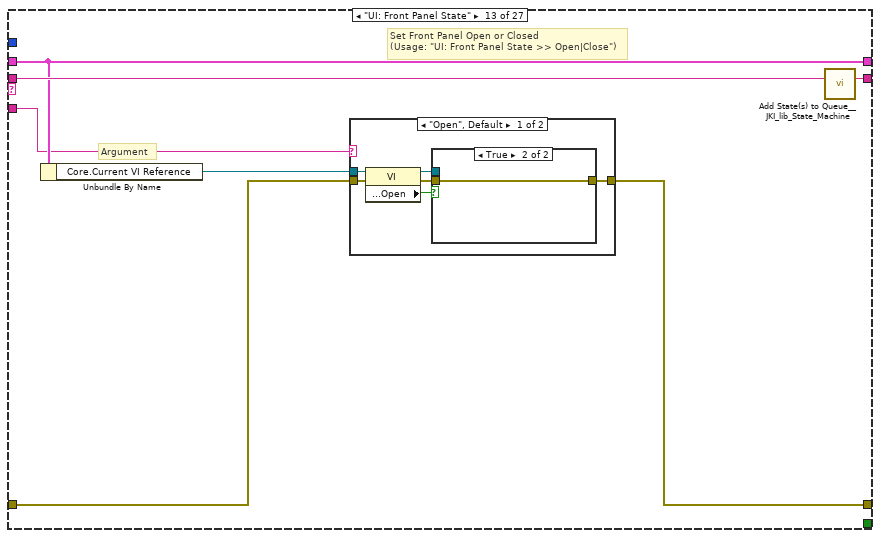
[diagram p18: hidden frame]
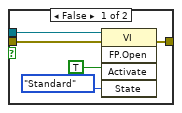
[diagram p19: hidden frame]
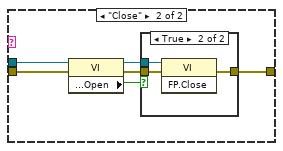
[diagram p20: hidden frame]
diagram:
  # "State Syntax:\nStateCategory: State >> Argument\nLine Terminator: Line feed\nExample:\nUI: Help >> About\n\nWhere \"UI\" is the state category\nWhere \"Help\" is the state\nWhere \"About\" is the argument\nOther Examples:\nApp Data: Initialize\nUI: Initialize\nHelp >> About\n\nCommenting:\nTo add a comment use \"//\" or \"#\" and all text to the right will be ignored\nCommenting Example:\nUI: Initialize // This initializes the UI\n# This whole line is a comment\n// Another comment line"
  # "copy this to create labels for wires"
  # "This controls the loop rate. -1 means wait forever in Event Structure"
  # "System_Label"
  n1 = call <vilib>:"Add State(s) to Queue__JKI_lib_State_Machine.vi"("State(s) in (\"\")"="Macro: Initialize") -> ("States Out"=w2:string)  [unwired: 14 in]
  n2 = while "JKI - String-Based Queued State Machine (Basic) v1.0" {
    shift-right: [w6] -> _
    shift-left: _ -> [w5]
    shift-right: [w9] -> _
    shift-left: _ -> [w3]
    shift-right: [w8] -> _
    shift-left: w2 -> [w10]
    stop <- w7 stop-if-true
    w4 = 50  # Timeout
    # "Template Copyright © 2015 JKI - http://jki.net/state-machine"
    n3 = call <vilib>:"Parse State Queue__JKI_lib_State_Machine.vi"("State Queue"=w10, "Error In (no error)"=w3) -> ("Remaining States"=w12:string, "Current State"=w13:string, "Arguments"=w11:string)  [unwired: 11 in]
    n4 = case shown="\"VISUALIZE: Graph Something\"" w13 {
      selector: w13 -> [_ _ w41 _ _ _ _ _ _ _ _ _ _ _ _ _ _ _ _ _ _ _ _ _ _ _ _]
      tunnel: w12 -> [w20 w40 w45 w63 w69 w74 w78 w83 w94 w98 w102 w108 w119 w145 w150 w160 w165 w176 w180 w203 w228 w232 w252 w265 w269 w281 w324]
      tunnel: w11 -> [_ _ _ _ _ _ _ _ _ _ _ w103 w113 _ _ _ _ _ _ _ _ _ _ _ _ _ _]
      tunnel: w5 -> [w18 w37 w43 w54 w66 w72 w75 _ w89 w95 w100 w106 w115 w142 w147 w157 w162 w173 w177 w197 w225 w229 w250 w262 w266 w271 w309]
      tunnel: [w17 w38 w47 w60 errorcluster {"status"=FALSE, "code"=0, "source"=""} ("error out") w71 w76 w80 w90 w96 w99 w104 w116 w143 w148 w158 w163 w174 w178 w189 w226 w230 w236 w263 w267 w279 w313] -> w9
      tunnel: w3 -> [w16 w38 w46 w60 w65 w71 w76 w80 w91 w96 w99 w105 w117 w143 w148 w158 w163 w174 w178 w200 w226 w230 w237 w263 w267 w279 w311]
      tunnel: [w19 w39 w44 w62 w68 w73 w77 w82 w93 w97 w101 w107 w118 w144 w149 w159 w164 w175 w179 w202 w227 w231 w251 w264 w268 w280 w323] -> w8
      tunnel: [_ _ _ _ _ TRUE _ _ _ _ _ _ _ _ _ _ _ _ _ _ _ _ _ _ _ _ _] -> w7
      tunnel: [w15 w37 w43 w61 w66 w72 w75 w79 w89 w95 w100 w106 w115 w142 w147 w157 w162 w173 w177 w196 w225 w229 w250 w262 w266 w270 w308] -> w6
      tunnel: w4 -> [w14 _ _ _ _ _ _ _ _ _ _ _ _ _ _ _ _ _ _ _ _ _ _ _ _ _ _]
      frame "", "Event Structure", "Idle" {
        # "executes when the state queue is empty"
        n5 = event shown="[2] Panel Close?" {
          selector: _ -> [_ _ _]
          dyn-events: _ -> [_ _ _]
          timeout: w14 -> [_ _ _]
          tunnel: w20 -> [w25 w30 w36]
          tunnel: [w24 w29 w35] -> w19
          tunnel: w18 -> [w22 w27 w33]
          tunnel: [w23 w28 w34] -> w17
          tunnel: w16 -> [w23 w28 w34]
          tunnel: [w22 w27 w33] -> w15
          event Timeout {
            n6 = event-data() -> ()  [unwired: 1 in, 1 out]
            n7 = call <vilib>:"Add State(s) to Queue__JKI_lib_State_Machine.vi"("State(s) in (\"\")"=w25, "State(s) at Back (\"\")"="//VISUALIZE: Cursor Things\nVISUALIZE: Graph Something" ("State(s) at Back (\"\")")) -> ("States Out"=w24:string)  [unwired: 13 in]
          }
          event "OK": Value Change {
            # "Exit Button Value Change (pressed) Event\n(this executes Macro: Exit to terminate the VI)"
            n8 = event-data() -> ()  [unwired: 1 in, 1 out]
            n9 = call <vilib>:"Add State(s) to Queue__JKI_lib_State_Machine.vi"("State(s) in Front (\"\")"="Macro: Exit", "State(s) in (\"\")"=w30) -> ("States Out"=w29:string)  [unwired: 13 in]
          }
          event Panel Close? {
            # "Discard the event because we'll close the front panel ourselves in Macro: Exit"
            # "Close Panel button (pressed) Event\n(this executes Macro: Exit to terminate the VI)"
            n10 = event-data() -> ()  [unwired: 1 in, 1 out]
            n11 = event-data("Discard?"=TRUE) -> ()  [unwired: 1 in, 1 out]
            n12 = call <vilib>:"Add State(s) to Queue__JKI_lib_State_Machine.vi"("State(s) in Front (\"\")"="Macro: Exit", "State(s) in (\"\")"=w36) -> ("States Out"=w35:string)  [unwired: 13 in]
          }
        }
      }
      frame "---------- Core ----------" {
        # "Do not put any code in this frame.\n(it is a separator no-op)"
        n13 = call <vilib>:"Add State(s) to Queue__JKI_lib_State_Machine.vi"("State(s) in (\"\")"=w40) -> ("States Out"=w39:string)  [unwired: 14 in]
      }
      frame Default {
        w50 = 42 items=["No error", "Argument error", "Memory is full", "Out of zone", "End of file", "File already open", "Generic file I/O error", "File not found", "File permission error", "Disk is full", "Duplicate path", "Too many files open", "System feature not enabled", "Resource file not found", "Cannot add resource", "Resource not found", "Image not found", "Image memory error", "Pen does not exist", "Config type invalid", "Config token not found", "Config parse error", "Config memory error", "Bad external code format", "Bad external code offset", "External code not present", "Null window", "Destroy window error", "Null menu", "Print aborted", "Bad print record", "Print driver error", "Windows error during printing", "Memory error during printing", "Print dialog error", "Generic print error", "Invalid device refnum", "Device not found", "Device parameter error", "Device unit error", "Cannot open device", "Device call aborted", "Generic error", "Cancelled by user", "Object ID too low", "Object ID too high", "Object not in heap", "Unknown heap", "Unknown object (invalid DefProc)", "Unknown object (DefProc not in table)", "Message out of range", "Invalid (null) method", "Unknown message", "Manager call not supported", "Bad address", "Network operation in progress", "Network operation timed out", "Connection is busy", "Network attribute not supported", "Network error", "Address in use", "System out of memory", "Connection aborted", "Connection refused", "Not connected", "Already connected", "Connection closed", "Initialization error (interapplication manager)", "Bad occurrence", "Wait on unbound occurrence handler", "Occurrence queue overflow", "Datalog type conflict", "Unused", "Unrecognized type (interapplication manager)", "Memory corrupt", "Failed to make temporary DLL", "Old CIN version", "Drag socket not found", "Failed to load drop-object", "Failed to register OLE object", "Failed to release OLE object", "Format specifier type mismatch", "Unknown format specifier", "Too few format specifiers", "Too many format specifiers", "Scan failed", "Newer CIN version", "Error converting to variant", "Runtime menu error", "Password tampered", "Variant attribute not found", "Incompatible variant data type", "Event data is not available", "Event Store is not present", "Occurrence is not found", "Event Queue is not created", "Event info is not available", "Refnum passed is NULL", "Error retrieving Class GUID", "Error retrieving CoClass GUID", "Error retrieving TypeLib GUID.", "Bad built application magic bytes.", "Specific driver is different from the specific driver associated with the Logical Name.", "There is no session opened to the class driver.", "Max Error", "MAX - Error with config objects", "MAX - Error loading configuration", "MAX - Group not supported"]
        # "Current State"
        # "Do not delete, rename, or modify this frame.\n(this is used to capture unhandled states and typos)"
        # "Handle mistyped state name (developer tool)"
        n14 = Format Into String(format string="Software Exception: Unhandled State \"%s\"." ("message"), error in=w46, w41) -> (resulting string=w49:string, error out=w48:errorcluster)  [unwired: 1 in]
        n15 = call <vilib>:"Error Cluster From Error Code.vi"("show call chain? (False)"=TRUE, "error in (no error)"=w48, "error message (\"\")"=w49, "error code (0)"=w50) -> ("error out"=w47:errorcluster)  [unwired: 5 in]
        n16 = call <vilib>:"Add State(s) to Queue__JKI_lib_State_Machine.vi"("State(s) in (\"\")"=w45) -> ("States Out"=w44:string)  [unwired: 14 in]
      }
      frame "Initialize Core Data" {
        # "Do not delete, rename, or modify this frame.\n(this is used to determine panel behavior on exit)"
        # "originally closed?"
        # "exe?"
        # "If panel starts closed or is an EXE, then close it when we exit"
        n17 = property class="VI"() -> ("Front Panel.Open"=w59:bool)  [unwired: 2 in, 2 out]
        n18 = property class="App"() -> ("App.Kind"=w58:T5)  [unwired: 2 in, 2 out]
        n19 = control-ref of="Current VI Reference"() -> (w52:refnum<vi>)
        n20 = Not(x=w59) -> (.not. x?=w56:bool)
        n21 = Equal?(x=w58, y=T5."Run Time System" ("Application:Kind")) -> (x = y?=w55:bool)
        n22 = Or(x=w56, y=w55) -> (x .or. y?=w53:bool)
        n23 = Bundle By Name(cluster=w54, "Core.Current VI Reference"=w52, "Core.Close Panel on Exit?"=w53) -> (w61:T7)
        n24 = call <vilib>:"Add State(s) to Queue__JKI_lib_State_Machine.vi"("State(s) in (\"\")"=w63) -> ("States Out"=w62:string)  [unwired: 14 in]
      }
      frame "Error Handler" {
        # "Unhandled Error -- Display it"
        # "Handle any errors here.\nYou can also output any states to clean-up after errors occur"
        # "Clear error"
        n25 = call <vilib>:"General Error Handler.vi"("error in (no error)"=w65) -> ()  [unwired: 10 in, 5 out]
        n26 = call <vilib>:"Add State(s) to Queue__JKI_lib_State_Machine.vi"("State(s) in Front (\"\")"="/* Post Error States", "State(s) in (\"\")"=w69) -> ("States Out"=w68:string)  [unwired: 13 in]
      }
      frame "Exit" {
        # "Do not put any code in this frame.\n(No errors that occur here will be handled.)"
        n27 = call <vilib>:"Add State(s) to Queue__JKI_lib_State_Machine.vi"("State(s) in (\"\")"=w74) -> ("States Out"=w73:string)  [unwired: 14 in]
      }
      frame "---------- DATA ----------" {
        # "Do not put any code in this frame.\n(It is a separator no-op. You can make a copy of this frame to create a new Data frame)"
        n28 = call <vilib>:"Add State(s) to Queue__JKI_lib_State_Machine.vi"("State(s) in (\"\")"=w78) -> ("States Out"=w77:string)  [unwired: 14 in]
      }
      frame "Data: Initialize" {
        w79 = T7 {"Core"={"Current VI Reference"=refnum, "Close Panel on Exit?"=FALSE}, "data value reference"=refnum, "Sweep Data Cluster"={"Vfast"=[], "Vslow"=[], "Vslowest"=[], "Comments"="", "Scan names"=[]}, "Cursor Info"={"Fast Index (Cursor X)"=[], "Slow Index (Cursor Y)"=0.0, "Slow Indices"=[], "Raw Cursor Position"={"X"=0.0, "Y"=0.0}, "Field / temp"=0}, "Scan names"=[]}  # State Wire IN
        w81 = T9 {"Current VI Reference"=refnum, "Close Panel on Exit?"=FALSE}  # Core
        # "do not delete - used by framework"
        # "Data names and types of shift register data are defined by this bundle."
        # "Initialize the shift-register data, here.\n(data names are defined by what you wire into the bundle function)"
        n29 = disable-structure shown="Disabled" {
          disable-tunnel: w81 -> [w86 _]
          frame Disabled {
            w85 = refnum<data-value> refnum  # DATA Cluster
            w88 = string[] ["DAQ_Vbg", "B", "B"]  # Scan names
            w87 = T10 {"Vfast"=[], "Vslow"=[], "Vslowest"=[], "Comments"="", "Scan names"=[]}  # Sweep Data Cluster
            n30 = Bundle("Core"=w86, "DATA Cluster"=w85, "Sweep Data Cluster"=w87, "Scan names"=w88) -> (w84)  [unwired: 1 in, 1 out]
          }
          frame Enabled {
          }
        }
        n31 = call <vilib>:"Add State(s) to Queue__JKI_lib_State_Machine.vi"("State(s) in (\"\")"=w83) -> ("States Out"=w82:string)  [unwired: 14 in]
      }
      frame "Data: Cleanup" {
        # "Cleanup any data and references, here.\n(this is called automatically, by the Macro: Exit)"
        n32 = Unbundle By Name(w89) -> ("Core.Current VI Reference"=w92:refnum<vi>)
        n33 = Close Reference(reference=w92, error in (no error)=w91) -> (error out=w90:errorcluster)
        n34 = call <vilib>:"Add State(s) to Queue__JKI_lib_State_Machine.vi"("State(s) in (\"\")"=w94) -> ("States Out"=w93:string)  [unwired: 14 in]
      }
      frame "---------- UI ----------" {
        # "Do not put any code in this frame.\n(It is a separator no-op. You can make a copy of this frame to create a new UI frame)"
        n35 = call <vilib>:"Add State(s) to Queue__JKI_lib_State_Machine.vi"("State(s) in (\"\")"=w98) -> ("States Out"=w97:string)  [unwired: 14 in]
      }
      frame "UI: Initialize" {
        # "Initialize the User Interface, here.\n(this is called automatically, by the Macro: Init)"
        n36 = call <vilib>:"Add State(s) to Queue__JKI_lib_State_Machine.vi"("State(s) in (\"\")"=w102) -> ("States Out"=w101:string)  [unwired: 14 in]
      }
      frame "UI: Cursor Set" {
        # "Argument"
        # "Set and Unset Cursor Busy.\n(Usage: \"UI: Cursor Set >> Busy|Idle\")"
        n37 = case shown="\"Idle\", Default" w103 {
          tunnel: w105 -> [w110 w112]
          tunnel: [w109 w111] -> w104
          frame "Idle", Default {
            n38 = call <vilib>:"Unset Busy.vi"("error in (no error)"=w110) -> ("error out"=w109:errorcluster)  [unwired: 10 in]
          }
          frame "Busy" {
            n39 = call <vilib>:"Set Busy.vi"("error in (no error)"=w112) -> ("error out"=w111:errorcluster)  [unwired: 9 in, 1 out]
          }
        }
        n40 = call <vilib>:"Add State(s) to Queue__JKI_lib_State_Machine.vi"("State(s) in (\"\")"=w108) -> ("States Out"=w107:string)  [unwired: 14 in]
      }
      frame "UI: Front Panel State" {
        # "Argument"
        # "Set Front Panel Open or Closed\n(Usage: \"UI: Front Panel State >> Open|Close\")"
        n41 = Unbundle By Name(w115) -> ("Core.Current VI Reference"=w114:refnum<vi>)
        n42 = case shown="\"Open\", Default" w113 {
          tunnel: w117 -> [w123 w136]
          tunnel: [w125 w137] -> w116
          tunnel: w114 -> [w124 w134]
          frame "Open", Default {
            n43 = property class="VI"(reference=w124, error in=w123) -> (reference out=w121:refnum<vi>, error out=w122:errorcluster, "Front Panel.Open"=w120:bool)
            n44 = case shown="True" w120 {
              tunnel: [w128 w131] -> w125
              tunnel: w122 -> [w127 w131]
              tunnel: w121 -> [w126 _]
              frame False {
                n45 = invoke class="VI" method="FP.Open"(reference=w126, error in=w127, "Activate"=TRUE, "State"=T6."Standard") -> (error out=w128:errorcluster)  [unwired: 1 in, 4 out]
              }
              frame True {
              }
            }
          }
          frame "Close" {
            n46 = property class="VI"(reference=w134, error in=w136) -> (reference out=w133:refnum<vi>, error out=w135:errorcluster, "Front Panel.Open"=w132:bool)
            n47 = case shown="True" w132 {
              tunnel: [w138 w141] -> w137
              tunnel: w135 -> [w138 w140]
              tunnel: w133 -> [_ w139]
              frame False {
              }
              frame True {
                n48 = invoke class="VI" method="FP.Close"(reference=w139, error in=w140) -> (error out=w141:errorcluster)  [unwired: 1 in, 2 out]
              }
            }
          }
        }
        n49 = call <vilib>:"Add State(s) to Queue__JKI_lib_State_Machine.vi"("State(s) in (\"\")"=w119) -> ("States Out"=w118:string)  [unwired: 14 in]
      }
      frame "---------- Macro ----------" {
        # "Do not put any code in this frame.\n(It is a separator no-op. You can make a copy of this frame to create a new Macro frame)"
        n50 = call <vilib>:"Add State(s) to Queue__JKI_lib_State_Machine.vi"("State(s) in (\"\")"=w145) -> ("States Out"=w144:string)  [unwired: 14 in]
      }
      frame "Macro: Initialize" {
        # "Initialization Macro\n(This is called once, when the VI starts)"
        n51 = call <vilib>:"Add State(s) to Queue__JKI_lib_State_Machine.vi"("State(s) in Front (\"\")"="Data: Initialize\nInitialize Core Data\nUI: Initialize\nUI: Front Panel State >> Open\nMacro: LOAD\nMacro: Visualize", "State(s) in (\"\")"=w150) -> ("States Out"=w149:string)  [unwired: 13 in]
      }
      frame "Macro: Exit" {
        # "Exit Macro\n(This is called once, when the VI exits)"
        n52 = Unbundle By Name(w157) -> ("Core.Close Panel on Exit?"=w156:bool)
        n53 = Select(t="UI: Front Panel State >> Close", s=w156, f="") -> (s? t:f=w153:string)
        n54 = call <vilib>:"Add State(s) to Queue__JKI_lib_State_Machine.vi"("State(s) in (\"\")"=w153, "State(s) at Back (\"\")"="Data: Cleanup\nExit") -> ("States Out"=w151:string)  [unwired: 13 in]
        n55 = call <vilib>:"Add State(s) to Queue__JKI_lib_State_Machine.vi"("State(s) in Front (\"\")"=w151, "State(s) in (\"\")"=w160) -> ("States Out"=w159:string)  [unwired: 13 in]
      }
      frame "Macro: LOAD" {
        # "Exit Macro\n(This is called once, when the VI exits)"
        n56 = call <vilib>:"Add State(s) to Queue__JKI_lib_State_Machine.vi"("State(s) in Front (\"\")"="LOAD: Load that .dat data" ("State(s) in Front (\"\")"), "State(s) in (\"\")"=w165) -> ("States Out"=w164:string)  [unwired: 13 in]
      }
      frame "Macro: VISUALIZE" {
        # "Skip or don't skip filtering step"
        # "Exit Macro\n(This is called once, when the VI exits)"
        n57 = Select(t="VISUALIZE: Apply SG Filter", s="Filter retrieved data? 2", f="") -> (s? t:f=w170:string)
        n58 = call <vilib>:"Add State(s) to Queue__JKI_lib_State_Machine.vi"("State(s) in Front (\"\")"="VISUALIZE: Initialize Cursor Graph\nVISUALIZE: Initialize Color Tables" ("State(s) in Front (\"\")"), "State(s) in (\"\")"=w170, "State(s) at Back (\"\")"="//VISUALIZE: Cursor Things\nVISUALIZE: Graph Something" ("State(s) at Back (\"\")")) -> ("States Out"=w169:string)  [unwired: 12 in]
        n59 = call <vilib>:"Add State(s) to Queue__JKI_lib_State_Machine.vi"("State(s) in Front (\"\")"=w169, "State(s) in (\"\")"=w176) -> ("States Out"=w175:string)  [unwired: 13 in]
      }
      frame "---------- LOAD ----------" {
        # "Template Separator\n(You can make a copy of, or modify, this frame)"
        n60 = call <vilib>:"Add State(s) to Queue__JKI_lib_State_Machine.vi"("State(s) in (\"\")"=w180) -> ("States Out"=w179:string)  [unwired: 14 in]
      }
      frame "LOAD: Load that .dat data" {
        # "scan data"
        # "Read .dat file"
        n61 = call "DataVIS_Read .DAT Data.vi"("error in (no error)"=w200, "file path (use dialog)"="file path (use dialog)") -> ("error out"=w189:errorcluster, "Array"=w198:T11)  [unwired: 8 in]
        n62 = Index Array(array=w198) -> (element=w199:T12)  [unwired: 1 in]
        n63 = Unbundle By Name(w199) -> ("IV-2T"=w188:cluster{dbl[], dbl[]}[][][], "IV"=w187:cluster{dbl[], dbl[]}[][][], "Vfast"=w195:dbl[][], "Vslow"=w194:dbl[], "Vslowest"=w193:dbl[], "Comments"=w192:string, "Scan names"=w190:string[])
        "Scan names" <- w190
        n64 = Bundle("Vfast"=w195, "Vslow"=w194, "Vslowest"=w193, "Comments"=w192, "Scan names"=w190) -> (w191:T10)  [unwired: 1 in]
        n65 = for {
          tunnel: w187 -> [w209] mode=indexing
          tunnel: [w208] -> w183 mode=indexing
          tunnel: [w207] -> w184 mode=indexing
          tunnel: w188 -> [w206] mode=indexing
          tunnel: [w205] -> w185 mode=indexing
          tunnel: [w204] -> w186 mode=indexing
          n66 = for {
            tunnel: w209 -> [w215] mode=indexing
            tunnel: [w214] -> w208 mode=indexing
            tunnel: [w213] -> w207 mode=indexing
            tunnel: w206 -> [w212] mode=indexing
            tunnel: [w211] -> w205 mode=indexing
            tunnel: [w210] -> w204 mode=indexing
            n67 = for {
              tunnel: w215 -> [w223] mode=indexing
              tunnel: [w224] -> w214 mode=indexing
              tunnel: [w221] -> w213 mode=indexing
              tunnel: w212 -> [w220] mode=indexing
              tunnel: [w217] -> w211 mode=indexing
              tunnel: [w216] -> w210 mode=indexing
              w219 = FALSE ("dy/dx vs x")
              w222 = TRUE ("dy/dx vs x")
              n68 = call <userlib>:"differential.vi"("Numeric"="Fit Points", "dy/dx vs x"=w222, "A vs B 2"=w220) -> ("A vs B 3"=w217:T13)  [unwired: 1 in]
              n69 = call <userlib>:"differential.vi"("Numeric"="Fit Points", "dy/dx vs x"=w219, "A vs B 2"=w220) -> ("A vs B 3"=w216:T13)  [unwired: 1 in]
              n70 = call <userlib>:"differential.vi"("Numeric"="Fit Points", "dy/dx vs x"=w219, "A vs B 2"=w223) -> ("A vs B 3"=w221:T13)  [unwired: 1 in]
              n71 = call <userlib>:"differential.vi"("Numeric"="Fit Points", "dy/dx vs x"=w222, "A vs B 2"=w223) -> ("A vs B 3"=w224:T13)  [unwired: 1 in]
            }
          }
        }
        n72 = Bundle("IV-2T"=w188, "IV"=w187, w186, w185, w184, w183) -> (w182:T14)  [unwired: 1 in]
        n73 = New Data Value Reference(data value=w182) -> (data value reference=w181:refnum<data-value>)  [unwired: 1 in, 1 out]
        n74 = Bundle By Name(cluster=w197, "data value reference"=w181, "Sweep Data Cluster"=w191, "Scan names"=w190) -> (w196:T7)
        n75 = call <vilib>:"Add State(s) to Queue__JKI_lib_State_Machine.vi"("State(s) in (\"\")"=w203) -> ("States Out"=w202:string)  [unwired: 14 in]
      }
      frame "LOAD: empty" {
        # "Your code here.\n(You can make a copy of, or modify, this frame)"
        n76 = call <vilib>:"Add State(s) to Queue__JKI_lib_State_Machine.vi"("State(s) in (\"\")"=w228) -> ("States Out"=w227:string)  [unwired: 14 in]
      }
      frame "---------- VISUALIZE ----------" {
        # "Template Separator\n(You can make a copy of, or modify, this frame)"
        n77 = call <vilib>:"Add State(s) to Queue__JKI_lib_State_Machine.vi"("State(s) in (\"\")"=w232) -> ("States Out"=w231:string)  [unwired: 14 in]
      }
      frame "VISUALIZE: Initialize Cursor Graph" {
        # "Template Separator\n(You can make a copy of, or modify, this frame)"
        n78 = Unbundle By Name(w250) -> ("Sweep Data Cluster.Vfast"=w243:dbl[][], "Sweep Data Cluster.Vslow"=w244:dbl[])  [unwired: 1 out]
        n79 = control-ref of="Cursor Graph"() -> (w234:refnum<vi>)
        n80 = local read "Scan names"() -> (w242:string[])
        n81 = Transpose 2D Array(2D array=w243) -> (transposed array=w249:dbl[][])
        n82 = for {
          tunnel: w249 -> [w258] mode=indexing
          tunnel: [w259] -> _ mode=indexing
          tunnel: w244 -> [w255]
          shift-right: [w256] -> w246
          shift-left: dbl[] [] -> [w257]
          shift-right: [w254] -> w245
          shift-left: dbl[] [] -> [w253]
          n83 = Build Array (concatenate)(w257, w258) -> (w256:dbl[])
          n84 = Build Array (concatenate)(w253, w255) -> (w254:dbl[])
          n85 = Bundle(w258, "Vslow"=w255) -> (w259:cluster{dbl[], "Vslow":dbl[]})  [unwired: 1 in]
        }
        n86 = Index Array(array=w242, index #2=1 ("index")) -> (element #1=w240:string, element #2=w239:string)  [unwired: 1 in]
        n87 = property on="Property Node" class="XYGraph (strict)"(reference=w234, error in=w237, "XScale.NameLbl.Text"=w240) -> (reference out=w233:refnum<vi>, error out=w238:errorcluster)
        n88 = property on="Property Node" class="XYGraph (strict)"(reference=w233, error in=w238, "YScale.NameLbl.Text"=w239) -> (error out=w236:errorcluster)  [unwired: 1 out]
        n89 = Bundle(w246, w245) -> (→"XY Graph 2":cluster{dbl[], dbl[]})  [unwired: 1 in]
        n90 = call <vilib>:"Add State(s) to Queue__JKI_lib_State_Machine.vi"("State(s) in (\"\")"=w252) -> ("States Out"=w251:string)  [unwired: 14 in]
      }
      frame "VISUALIZE: Initialize Color Tables" {
        # "#TODO:"
        # "Set color tables"
        # "Template Separator\n(You can make a copy of, or modify, this frame)"
        n91 = Reverse 1D Array(array="color scale") -> (reversed array=w261:u32[])
        n92 = call <userlib>:"Make Color Table.vi"("Array"=w261) -> ()  [unwired: 1 in, 4 out]
        n93 = call <vilib>:"Add State(s) to Queue__JKI_lib_State_Machine.vi"("State(s) in (\"\")"=w265) -> ("States Out"=w264:string)  [unwired: 14 in]
      }
      frame "VISUALIZE: Apply SG Filter" {
        # "NOT IMPLEMENTED YET\n#TODO: this"
        # "Template Separator\n(You can make a copy of, or modify, this frame)"
        n94 = call <vilib>:"Add State(s) to Queue__JKI_lib_State_Machine.vi"("State(s) in (\"\")"=w269) -> ("States Out"=w268:string)  [unwired: 14 in]
      }
      frame "VISUALIZE: Cursor Things" {
        # "trash if this all gets put into In-place element structure"
        # "#TODO: work out this state logic, for now just repeat\n'case 3' cursor things and graph something"
        # "Template Separator\n(You can make a copy of, or modify, this frame)"
        n95 = Unbundle By Name(w271) -> ("Sweep Data Cluster.Vfast"=w278:dbl[][], "Sweep Data Cluster.Vslow"=w277:dbl[], "Sweep Data Cluster.Vslowest"=w276:dbl[])
        n96 = disable-structure shown="Disabled" {
          disable-tunnel: w278 -> [w295 _]
          disable-tunnel: w277 -> [w294 _]
          disable-tunnel: w276 -> [w293 _]
          disable-tunnel: [w292 _] -> w275
          disable-tunnel: [w291 _] -> w274
          disable-tunnel: [w290 _] -> w273
          disable-tunnel: [w289 _] -> w272
          frame Disabled {
            n97 = Index Array(array=w293) -> (element=w283:dbl, index=w285:i32)
            n98 = Array Size(array=w293) -> (size(s)=w288:i32)
            n99 = call "DataVIS_Get_Cursor_Indices.vi"("Vslow"=w294, "Vfast"=w295) -> ("Slow Indices"=w290:dbl[], "Slow Index (Cursor Y)"=w291:dbl, "Fast Index (Cursor X) (IDK why it's an array)"=w292:dbl[], "Raw Cursor Position"=w289:T8, "Cursor Graph"=w286:refnum<vi>)  [unwired: 4 in, 1 out]
            n100 = Decrement(x=w288) -> (x-1=w287:i32)
            n101 = Unbundle By Name(w289) -> ("Y"=w282:dbl)  [unwired: 1 out]
            n102 = property on="Property Node" class="Slide (strict)"("Scale.Maximum"=w287) -> (reference=w284:refnum<vi>)  [unwired: 1 in, 2 out]
          }
          frame Enabled {
          }
        }
        n103 = disable-structure shown="Disabled" {
          frame Disabled {
            n104 = local read "side points 4Ttemp"() -> (w305:i32)
            n105 = local read "side points 2Ttemp"() -> (w306:i32)
            n106 = local read "side points 2T 2"() -> (w307:i32)
            n107 = local read "side points 4T 2"() -> (w304:i32)
            n108 = Not Equal?(x=w305, y=w304) -> (x != y?=w303:bool)
            n109 = Not Equal?(x=w307, y=w306) -> (x != y?=w302:bool)
            n110 = Or(x=w303, y=w302) -> (x .or. y?=w301:bool)
            n111 = Select(t=2, s=w301, f=3) -> (s? t:f=w296:i32)
            n112 = Select(t=4, s="stop", f=w296) -> ()  [unwired: 1 out]
          }
          frame Enabled {
          }
        }
        n113 = Bundle By Name(cluster=w271, "Cursor Info.Fast Index (Cursor X)"=w275, "Cursor Info.Slow Index (Cursor Y)"=w274, "Cursor Info.Slow Indices"=w273, "Cursor Info.Raw Cursor Position"=w272) -> (w270:T7)
        n114 = call <vilib>:"Add State(s) to Queue__JKI_lib_State_Machine.vi"("State(s) in (\"\")"=w281) -> ("States Out"=w280:string)  [unwired: 14 in]
      }
      frame "VISUALIZE: Graph Something" {
        # "#TODO: if it's slow, keep the main looping INSIDE this"
        n115 = Unbundle By Name(w309) -> ("data value reference"=w310:refnum<data-value>, "Sweep Data Cluster"=w322:T10, "Cursor Info"=w318:T15, "Scan names"=w312:string[])
        n116 = Unbundle By Name(w318) -> ("Fast Index (Cursor X)"=w317:dbl[], "Slow Index (Cursor Y)"=w316:dbl, "Slow Indices"=w315:dbl[], "Raw Cursor Position"=w314:T8)
        n117 = Unbundle By Name(w322) -> ("Vfast"=w321:dbl[][], "Vslow"=w320:dbl[], "Vslowest"=w319:dbl[])
        n118 = in-place {
          in-place-border: w321 -> [_]
          in-place-border: w320 -> [_]
          in-place-border: w319 -> [_]
          in-place-border: w317 -> [_]
          in-place-border: w316 -> [_]
          in-place-border: w315 -> [_]
          in-place-border: w314 -> [_]
          in-place-border: [w330] -> w313
          in-place-border: w312 -> [_]
          in-place-border: w311 -> [w338]
          in-place-border: w309 -> [w333]
          in-place-border: [w328] -> w308
          # "This is where all the plots and things go... somehow"
          # "update cursor info"
          n119 = in-place-dvr #1(w310) -> (w326:T16)  [unwired: 1 out]
          n120 = control-ref of="Cursor Graph"() -> (w332:refnum<vi>)
          n121 = local read "Field/Temperature"() -> (w337:i32)
          n122 = control-ref of="Field/Temperature"() -> (w336:refnum<vi>)
          n123 = call "DataVIS_Update_Cursor.vi"("Field/Temperature 2"=w336, "error in (no error)"=w338, "Cursor Graph"=w332, "Field / temp"=w337, "State Wire IN"=w333) -> ("error out"=w331:errorcluster, "Field"=→"Field":dbl, "slowest"=→"slowest":dbl, "State Wire OUT"=w329:T7)  [unwired: 3 in]
          n124 = case shown="\"2 terminal G vs V\"" "Tab Control" {
            tunnel: w331 -> [_ w343 _ _ _ _ w368 _ _ _ _]
            tunnel: [_ w342 _ _ _ _ _ _ _ _ _] -> w330
            tunnel: w329 -> [_ w341 _ _ _ _ w367 _ _ _ _]
            tunnel: [_ w340 _ _ _ _ w369 _ _ _ _] -> w328
            tunnel: w326 -> [_ _ _ _ _ _ w370 _ _ _ _]
            tunnel: "derivative bin size (also for 2T)" -> [_ _ _ _ _ _ w357 _ _ _ _]
            frame "Device ", Default {
            }
            frame "Data generation" {
              n125 = call "DataVIS_FormatIntensityScales.vi"("error in (no error)"=w343, "Decimate Controls"="Decimate Controls", "State Wire IN"=w341) -> ("error out"=w342:errorcluster, "State Wire OUT"=w340:T7)  [unwired: 6 in, 1 out]
              n126 = call "DataVIS_Decimate+Fill_Intensity_Plot.vi"() -> ()  [unwired: 8 in, 4 out]
            }
            frame "Vary Vfast" {
            }
            frame "Vary Vslow" {
            }
            frame "Vary Fields" {
            }
            frame "4 terminal G vs V" {
            }
            frame "2 terminal G vs V" {
              n127 = Unbundle By Name(w370) -> ("dI/dV 2T"=w366:cluster{dbl[], dbl[]}[][][])
              n128 = control-ref of="2term Intensity 2"() -> (w350:refnum<vi>)
              n129 = control-ref of="2 term trans"() -> (w351:refnum<vi>)
              n130 = call "DataVIS_Select_Intensity_Array.vi"("error in (no error)"=w368, "dI/dV 2T 2"=w366, "State Wire IN"=w367) -> ("error out"=w365:errorcluster, "Intensity Array OUT"=w363:cluster{dbl[], dbl[]}[], "State Wire OUT"=w361:T7)  [unwired: 6 in]
              n131 = call "DataVIS_Decimate+Fill_Intensity_Plot.vi"("Log Scale (T)"="Log scale? 4", "error in (no error)"=w365, "fake point value"="fake point value 2", "Decimate Controls"="Decimate Controls 2", "X and Y Arrays to decimate"=w363) -> ("error out"=w364:errorcluster, "Decimated X values"=w356:dbl[], "Arr of Y arrays (intensity info)"=w345:dbl[][])  [unwired: 3 in, 1 out]
              "2term Intensity 2" <- w345
              n132 = Bundle("2term Intensity 2"=w350, "2 term trans"=w351) -> (w352:T17)  [unwired: 1 in]
              n133 = call "DataVIS_FormatIntensityScales.vi"("error in (no error)"=w364, "Control References"=w352, "Decimate Controls"="Decimate Controls 2", "State Wire IN"=w361) -> ("error out"=w358:errorcluster, "Vfast values"=w355:dbl[], "State Wire OUT"=w369:T7)  [unwired: 5 in]
              n134 = call "transcond_intensity_v2.vi"("derivative bin size"=w357, "Conductance"=w345) -> ("Transconductance"=w344:dbl[][])  [unwired: 9 in]
              "2 term trans" <- w344
              n135 = call "DataVIS_LineCuts.vi"("Intensity Plot"=w350, "e^2/h?"="e^2/h?", "error in (no error)"=w358, "Vfast values"=w355, "Decimated X values"=w356, "Arr of Y arrays (intensity info)"=w345) -> ("error out"=w354:errorcluster, "X line cut"=→"X line cut":cluster{dbl[], dbl[]}, "Y line cut"=→"Y line cut":cluster{"Vfast":dbl[], dbl[]})  [unwired: 3 in]
              n136 = call "DataVIS_LineCuts.vi"("Intensity Plot"=w351, "e^2/h?"="e^2/h?", "error in (no error)"=w354, "Vfast values"=w355, "Decimated X values"=w356, "Arr of Y arrays (intensity info)"=w344) -> ("X line cut"=→"2term trans X line cut":cluster{dbl[], dbl[]}, "Y line cut"=→"2term trans Y line cut":cluster{"Vfast":dbl[], dbl[]})  [unwired: 3 in, 1 out]
            }
            frame "4 terminal R vs I" {
            }
            frame "2 terminal R vs I" {
            }
            frame "3D" {
            }
            frame "Whatever" {
            }
          }
          n137 = in-place-dvr #1(w326) -> ()  [unwired: 2 out]
        }
        n138 = call <vilib>:"Add State(s) to Queue__JKI_lib_State_Machine.vi"("State(s) in (\"\")"=w324) -> ("States Out"=w323:string)  [unwired: 14 in]
      }
    }
  }
